vi "Magnetic_Scale_Writing.vi"() -> ()   [LabVIEW 2013]
uses:
  <vilib>/event_ctls.llb/eventvkey.ctl
  Global_Not-Aus.vi
  Global_Start_Stop_Einzelschritt.vi
  <vilib>/Utility/file.llb/Write To Spreadsheet File (DBL).vi
  <vilib>/Instr/_visa.llb/VISA Configure Serial Port (Instr).vi
  <vilib>/Utility/file.llb/Read From Spreadsheet File (string).vi
panel:
  in  "RON settings":T1={"RON Affected axes"=[], "Reference mode"=[], "Check FRF?"=TRUE}
  out "error out 8":errorcluster
  out "error out 4":errorcluster
  out "read buffer":string
  out "error out 7":errorcluster
  out "error out 6":errorcluster
  out "error out 5":errorcluster
  in  "error in 4":errorcluster
  in  "write buffer":string="raw_alls"
  in  "Schritte oder mm (mm)":u16(ring) items=["Schritte", "mm"]
  in  "write ED33 2":string="z\\r"
  in  "write ED33":string="Z\\r"
  out "Diff":i64
  out "Ref_Steps":i64
  out "ED33_pos":i64
  out "ED33_array":string[](array[string])
  out "error out 3":errorcluster
  out "error out 2":errorcluster
  out "error out":errorcluster
  in  "error in":errorcluster
  in  "Tab Control":enum32{"Page 2"}(tab)
  in  "Main Tab":enum32{"Page 1", "Page 2"}(tab)
  out "SensorStage - Zaxis":dbl[](array[numeric]) format="%.6f"
  out "Steps":dbl
  out "Current Sequence":string[](array[string])
  in  "Clear Sequence":bool
  in  "Load Sequence":bool
  out "Sequence":string[][](array[string])
  in  "File  Select":path
  in  "Activate Sequence?":bool
  in  "Multiple Control":T2(tab)
  out "P6":dbl[](array[numeric])
  out "P5":dbl[](array[numeric])
  out "P4":dbl[](array[numeric])
  out "P3":dbl[](array[numeric])
  out "P7":dbl[](array[numeric])
  out "P2":dbl[](array[numeric])
  out "P1":dbl[](array[numeric])
  out "P8":dbl[](array[numeric])
  out "P9":dbl[](array[numeric])
  out "P10":dbl[](array[numeric])
  in  "Z axis":enum16{"Up", "Down"}(ring)
  in  "Y axis":enum16{"Forward", "Backward"}(ring)
  in  "X axis":enum16{"Left", "Right"}(ring)
  in  "Move Steps":bool
  in  "Steps(mm)":dbl[](array[numeric]) min=0.0
  in  "Go To":bool
  in  "Position":T3(ring)
  in  "Save":bool
  in  "Reset All":bool
  in  "Reset":bool
  in  "Import":bool
  in  "Export":bool
  in  "File Path":path=path "Y:/01_Projekte/EPN93031_Schreibplatz/8_Konstruktionsunterlagen/8.5_Software/COPY_KOSY Steuerung LabVIEW/1.New_Code_2014_2015/New_Scripts/1Poletab_position_Ghead.txt"
  out "Speed":dbl(knob) scale=0.0..10.0
  in  "Port for KOSY3":refnum<visa-resource-name>="COM2"
  in  "Port for Powersupply":refnum<visa-resource-name>="COM3"
  in  "Port for Write Head":refnum<visa-resource-name>="COM4"
  in  "Port for ED33":refnum<visa-resource-name>="COM7"
  in  "Port for Sensors":refnum<visa-resource-name>="COM6"
  in  "X,Y,Z Value Limits":T4={"mm Xmin "=0.0, "mm Xmax "=100.0, " mm Ymin "=0.0, "mm Ymax "=267.9, " mm Zmin"=0.0, "mm Zmax "=108.0, "Schritte oder mm Umin (0)"=0.0, "Schritte oder mm Umax (0)"=0.0, "Schritte oder mm Cmin (0)"=0.0, "Schritte oder mm Cmax (0)"=0.0, "Schritte oder mm Amin (0)"=0.0, "Schritte oder mm Amax (0)"=0.0, "Schritte oder mm Bmin (0)"=0.0, "Schritte oder mm Bmax (0)"=0.0}
  out "Error Out":errorcluster caption="error out"
  in  "Error In":errorcluster caption="error in"
  out "Movement":T5={"Axis"=36, "Direction(To/From)"=0, "Speed in mm/s\n (5)[0,025-20]"=5.0, "IV6"=FALSE} {"Direction(To/From)" items=["vom Endschalter weg", "zum Endschalter hin"]; "Speed in mm/s\n (5)[0,025-20]" min=0.025 max=20; "Axis" items=["X-Achse"=36, "Y-Achse"=37, "Z-Achse"=38, "U-Achse"=63]}
  out "Keyboard Press Display":cluster{"Speed(+/-)":i16, "Movement":T6}
  in  "Y_Axis_Select":string(combo)="PI"
  in  "Read Sensor":bool
  in  "Pole Pitch":string(combo)
  in  "Move WithRef":bool
  in  "Sensor Box":string(combo)="MLS5000"
  in  "Sensors Active?":bool
  in  "ED33 Active?":bool
  out "Sensor":cluster{i32, i32}(graph)
  in  "Count":dbl
  in  "Move & Measure":bool
  in  "Clear Sensor Readings":bool
  out "ED33_output":string[][](array[string])
  out "Sensor_output":string[][](array[string])
  out "ED33":i32[](graph)
  out "Sensor Output":string[](array[string])
  out "current time":timestamp
  in  "Move Rel Y":bool
  in  "Stop YaxisStage":bool caption="Stop Yaxis Stage"
  in  "Position to move-Y":dbl[](array[numeric]) format="%.6f"
  in  "Move Abs Y":bool
  in  "Steps to move-Y":dbl[](array[numeric]) format="%.6f"
  in  "System no.Y":i32=2 min=1 step=1
  in  "Axes to move Y":string[](array[string])=["1"]
  out "Ref. Position Y":dbl[](array[numeric]) format="%.6f"
  out "Serial Number Y":string="0145500519"
  in  "Interface Y":u16(ring)=2 items=["RS232", "RS232 DaisyChain", "USB", "USB_DaisyChain"]
  in  "Stop Sensor Stage":bool
  in  "Move Rel S":bool
  in  "Move Abs S":bool
  in  "System no. S":i32=1 min=1 step=1
  in  "Interface S":u16(ring)=2 items=["RS232", "RS232 DaisyChain", "USB", "USB_DaisyChain"]
  in  "Axes to move S":string[](array[string])=["1"]
  out "Serial Number S":string="0135500035"
  out "Ref. Position S":dbl[](array[numeric]) format="%.6f"
  in  "Position to move-S":dbl[](array[numeric]) format="%.6f"
  in  "Steps to move-S":dbl[](array[numeric]) format="%.6f"
  out "Operation Done":string="Initialise"
  out "Current Status":string="Initialise"
  out "Moving":bool
  out "Stopped":bool
  in  "Stop Program":bool
  in  "Home Position":bool
  out "Current Cordinates":T7 {"Schritte B" format="%#.4g"; "Schritte A" format="%#.4g"; "Schritte C" format="%#.4g"; "Schritte U" format="%#.4g"; "Z axis" format="%#.4g"; "Y axis" format="%#.4g"; "X axis" format="%#.4g"}
  out "Yaxis Stage":dbl[](array[numeric]) format="%.6f"
  # "Instructions\n                                              Manual Control\n1. First run PIMikroMove to reference C-863 motor. \n2. Run the program.\n3. Select 'Initialise' to start the program from first \n     or 'Continue' to continue the ongoing process.\n4. Select 'Normal Operation'.\n\nPolestrip Positions\n1. If positions are already saved, select the corresponding \n    file in 'File Path' and then click 'Import' to get the corresponding\n    positions displayed on the front panel. \n2. Set the 'Speed' using (+/-) for the movement.\n3. Select a position from the dropdown 'Position'and click 'Go To'.\n    Else, \n1. Set the 'Speed' using (+/-) for the movement.\n2. Set the length for movement in 'Steps(mm)'  in corresponding \n    axis and also the direction of travel in the selected axis. \n    Then press 'Move'.\n3. Once desired position is reached, select a position from the \n    dropdown 'Position' and click 'Save'.\n4. Once all positions are saved in front panel, select the file  to be \n     saved in 'File Path' and click 'Export' to save positions to a text file.\n5. Select a position from the dropdown 'Position' and \n    Click 'Reset' to clear individual position.\n6. Click 'Reset All' to clear all positions.\n \nSensor Readings\nContinuous measurement\n1.Activate the sensor to be read from 'Read Sensors' tab.\n2.Set the length for movement in 'Steps(mm)' in corresponding \n    axis and also the direction of travel in the selected axis. \n    Then press 'Move'.\nMove and Measure\n1. Activate the sensor to be read from 'Read Sensors' tab.\n2.Set 'Count' to the number of times to measure.\n2.Set the length for movement in 'Steps(mm)' in corresponding \n    axis and also the direction of travel in the selected axis. \n    Then press 'Move Measure'.\n\n1. Click 'Clear' in 'Read Sensors' tab to clear the sensor readings.\n\n                                          Automatic Execution\n1. First run PIMikroMove to reference C-863 motor. \n2. Run the program.\n3. Select 'Initialise' to start the program from first \n     or 'Continue' to continue the ongoing process.\n4. Select 'Normal Operation'.\n5. Select the corresponding file in 'File Select' and then click 'Load' \n    to get the corresponding codes in 'Sequence' .\n6. Click 'Clear' to clear sequence.\n7. Click 'Activate Sequence?' to run the automatic execution. \n\n                                                       General\n1. Click 'Stop Program' to stop the running program.\n2. Click 'Home Position' to take the write head to (0,0,0)."
  # "Write & Read Apparatus ( Control Panel )"
  # "Polestrip Positions"
  # "Com port info"
  # "Waveform Dispaly"
  # "Stage Move - Abs"
  # "Stage Move - Rel"
  # "Stage Move - Abs"
  # "Stage Move - Rel"
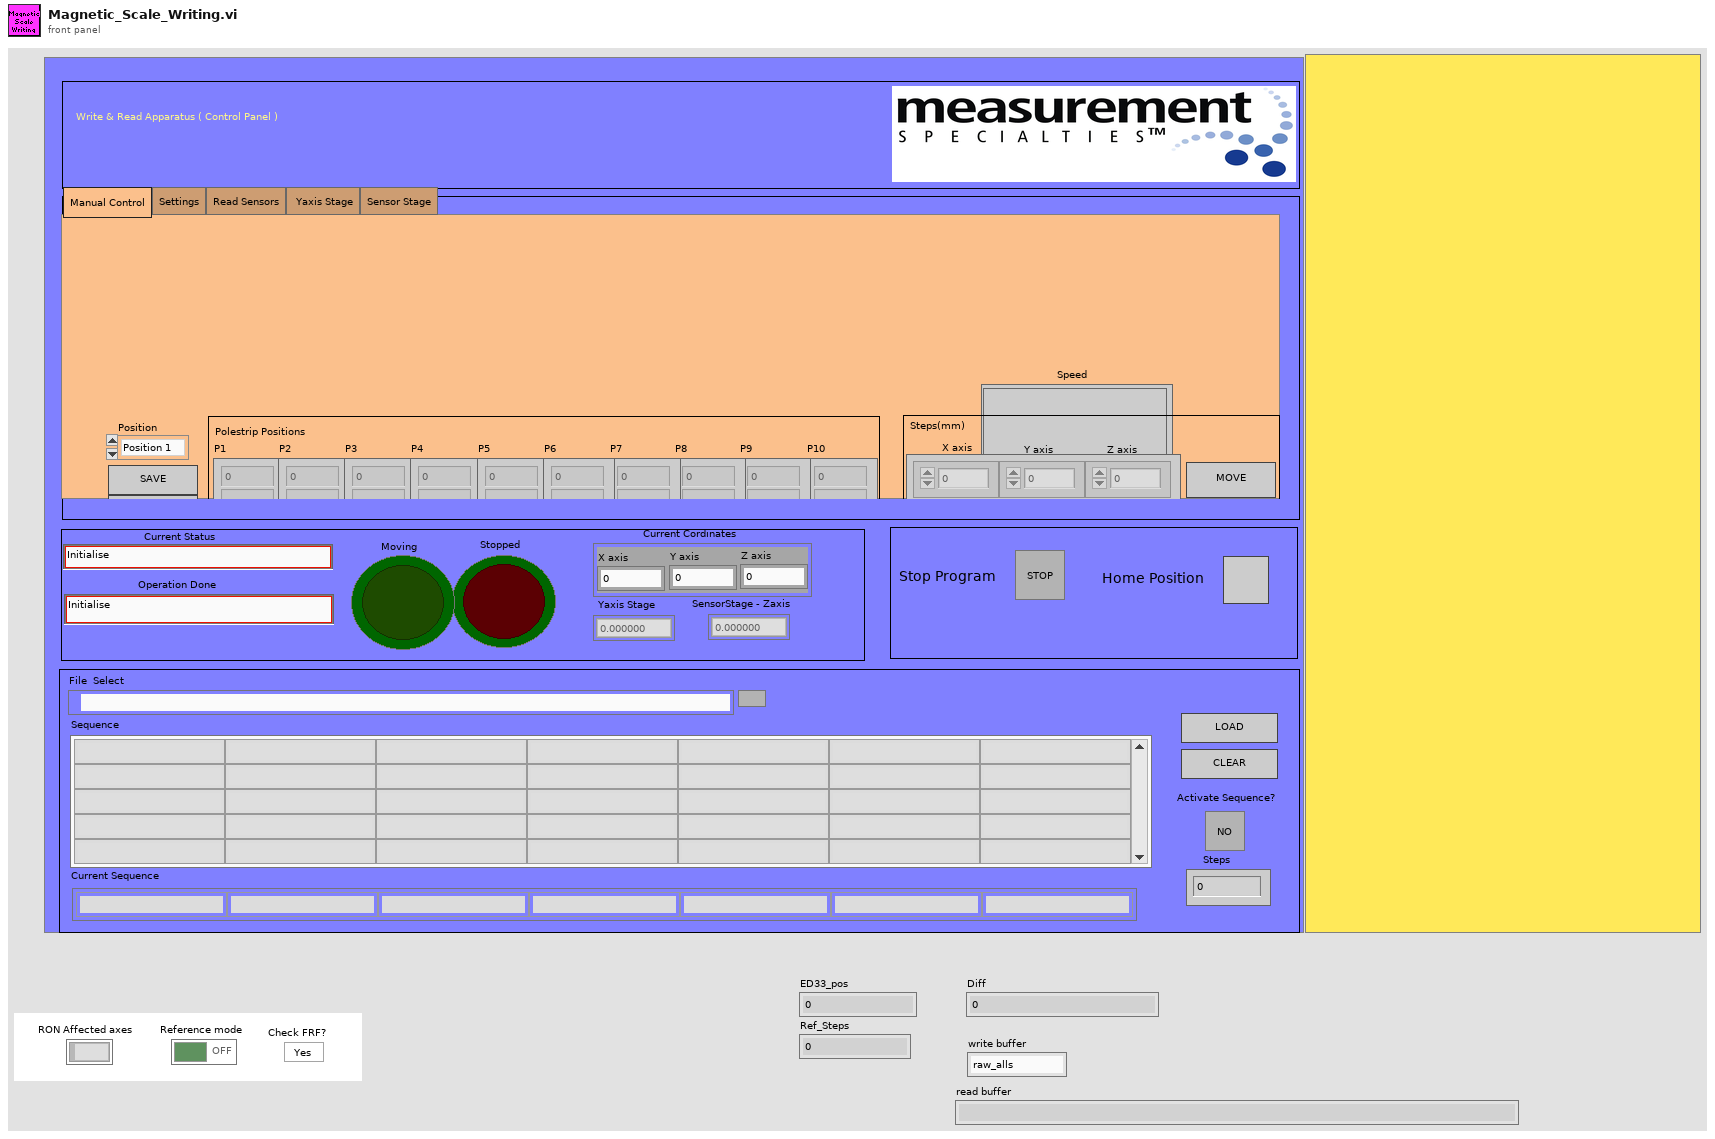
[diagram p1: front panel]
types:
  T1 = cluster{"RON Affected axes":string[], "Reference mode":bool[], "Check FRF?":bool}
  T2 = enum32{"Manual Control", "Settings", "Read Sensors", " Yaxis Stage", "Sensor Stage"}
  T3 = enum16{"Position 1", "Position 2", "Position 3", "Position 4", "Position 5", "Position 6", "Position 7", "Position 8", "Position 9", "Position 10"}
  T4 = cluster{"mm Xmin ":sgl, "mm Xmax ":sgl, " mm Ymin ":sgl, "mm Ymax ":sgl, " mm Zmin":sgl, "mm Zmax ":sgl, "Schritte oder mm Umin (0)":sgl, "Schritte oder mm Umax (0)":sgl, "Schritte oder mm Cmin (0)":sgl, "Schritte oder mm Cmax (0)":sgl, "Schritte oder mm Amin (0)":sgl, "Schritte oder mm Amax (0)":sgl, "Schritte oder mm Bmin (0)":sgl, "Schritte oder mm Bmax (0)":sgl}
  T5 = cluster{"Axis":u8, "Direction(To/From)":u8, "Speed in mm/s\n (5)[0,025-20]":sgl, "IV6":bool}
  T6 = typedef "eventvkey.ctl" = enum16{"ASCII", "Enter", "Return", "Shift", "Ctrl", "Alt", "Cmd", "Opt", "Caps", "NumLock", "Clear", "Break", "Up", "Down", "Left", "Right", "Insert", "Delete", "Home", "End", "PageUp", "PageDown", "Escape", "Help", "Pause", "ScrollLock", "F1", "F2", "F3", "F4", "F5", "F6", "F7", "F8", "F9", "F10", "F11", "F12", "F13", "F14", "F15", "F16", "F17", "F18", "F19", "F20", "F21", "F22", "F23", "F24", "Play", "VolumeUp", "VolumeDown", "Mute", "Two Byte Char"}
  T7 = cluster{"X axis":sgl, "Y axis":sgl, "Z axis":sgl, "Schritte U":sgl, "Schritte C":sgl, "Schritte A":sgl, "Schritte B":sgl}
  T8 = cluster{"Geschwindigkeit X in mm/s\n(5) [0,025-15]":sgl, "Geschwindigkeit Y in mm/s\n(5) [0,025-15]":sgl, "Geschwindigkeit Z in mm/s\n(5) [0,025-15]":sgl, "GeschwindigkeitU in mm/s\n(5) [0,025-15]":sgl}
  T9 = cluster{"Schritte X":sgl, "Schritte Y":sgl, "Schritte Z":sgl, "Schritte U":sgl, "Schritte C":sgl, "Schritte A":sgl, "Schritte B":sgl}
  T10 = cluster{"[0]":dbl, "[1]":dbl, "[2]":dbl, "[3]":dbl, "[4]":dbl, "[5]":dbl, "[6]":dbl, "[7]":dbl, "[8]":dbl}
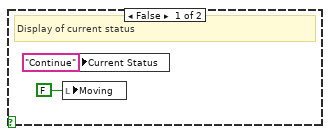
[diagram p5: hidden frame]
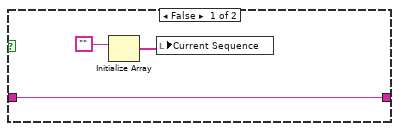
[diagram p6: hidden frame]
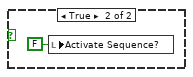
[diagram p7: hidden frame]
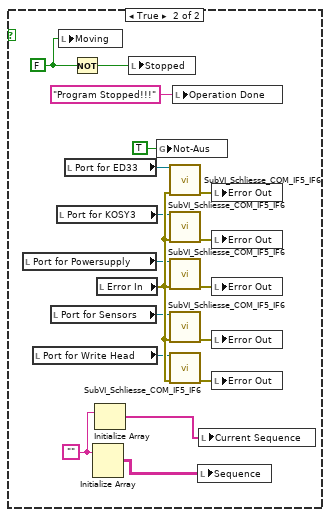
[diagram p8: hidden frame]
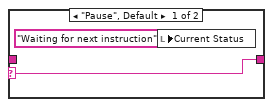
[diagram p9: hidden frame]
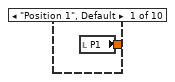
[diagram p11: hidden frame]
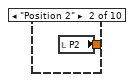
[diagram p12: hidden frame]
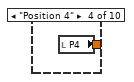
[diagram p13: hidden frame]
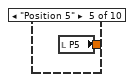
[diagram p14: hidden frame]
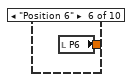
[diagram p15: hidden frame]
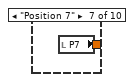
[diagram p16: hidden frame]
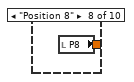
[diagram p17: hidden frame]
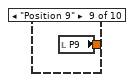
[diagram p18: hidden frame]
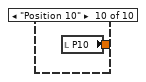
[diagram p19: hidden frame]
diagram:
  n1 = stacked-sequence {
    tunnel: [_ w29] -> w1
    frame #0 {
      w6 = i64 0 ("ED33_pos")
      w8 = 0.0 ("Speed")
      w4 = "" ("element")
      w9 = dbl[] [0.0, 0.0, 0.0] ("P1")
      w2 = FALSE ("Moving")
      # "Start Options - The program starts in this window with an initilialisation. It sets the current status, set all the corresponding booleans to 'False' and the passes on the flow to the next window for further initialisation of the KOSY3 platform and other processes."
      n2 = local read "Error In"() -> (w15:errorcluster)
      n3 = call "Start"("error in (no error)"=w15) -> ("Initialise"=w13:bool, "error out"=w14:errorcluster)  [unwired: 17 in]
      n4 = local write "Error Out"(w14) -> ()
      n5 = case shown="True" w13 {
        frame False {
        }
        frame True {
          n6 = local read "Port for KOSY3"() -> (w18:refnum<visa-resource-name>)
          n7 = local read "Error In"() -> (w17:errorcluster)
          n8 = call "SubVI_Schliesse_COM_IF5_IF6.vi"("VISA resource name in"=w18, "error in"=w17) -> ("error out"=w16:errorcluster)  [unwired: 13 in]
          n9 = local write "Error Out"(w16) -> ()
        }
      }
      n10 = case shown="True" w13 {
        frame False {
          # "Display of current status"
          n11 = local write "Moving"(FALSE ("Stopped")) -> ()
          n12 = local write "Current Status"("Continue") -> ()
        }
        frame True {
          w26 = FALSE ("Stopped")
          # "Display of current status"
          n13 = local write "Current Status"("Initialise") -> ()
          n14 = local write "Stopped"(w26) -> ()
          n15 = Not(x=w26) -> (.not. x?=w27:bool)
          n16 = local write "Moving"(w27) -> ()
        }
      }
      n17 = case shown="True" w13 {
        frame False {
        }
        frame True {
          w22 = u16 0 items=["vom Endschalter weg", "zum Endschalter hin"]
          w23 = u16 36 items=["x-axis"=36, "y-axis"=37, "z-axis"=38]
          # "Initialy setting the boolean in the cluster to False"
          n18 = Bundle(w23, w22, 0.0, FALSE) -> (w19:cluster{u16, u16, dbl, bool})  [unwired: 1 in]
          n19 = local write "Movement"(w19) -> ()
        }
      }
      n20 = local write "Steps(mm)"(w9) -> ()
      n21 = local write "Save"(w2) -> ()
      n22 = local write "Reset"(w2) -> ()
      n23 = local write "Go To"(w2) -> ()
      n24 = local write "Export"(w2) -> ()
      n25 = local write "Move Abs S"(w2) -> ()
      n26 = local write "Move Rel S"(w2) -> ()
      n27 = local write "Stop YaxisStage"(w2) -> ()
      n28 = local write "Move Abs Y"(w2) -> ()
      n29 = local write "Move Rel Y"(w2) -> ()
      n30 = global write "Global_Not-Aus.vi" "Not-Aus"(w2) -> ()
      n31 = local write "Stop Program"(w2) -> ()
      n32 = local write "Stopped"(w2) -> ()
      n33 = local write "Moving"(w2) -> ()
      n34 = local write "Load Sequence"(w2) -> ()
      n35 = local write "Clear Sequence"(w2) -> ()
      n36 = local write "Activate Sequence?"(w2) -> ()
      n37 = local write "Reset All"(w2) -> ()
      n38 = local write "Move WithRef"(w2) -> ()
      n39 = local write "Import"(w2) -> ()
      n40 = local write "Move Steps"(w2) -> ()
      n41 = local write "Sensors Active?"(w2) -> ()
      n42 = local write "ED33 Active?"(w2) -> ()
      n43 = local write "Clear Sensor Readings"(w2) -> ()
      n44 = local write "Move & Measure"(w2) -> ()
      n45 = local write "Stop Sensor Stage"(w2) -> ()
      n46 = local write "Read Sensor"(w2) -> ()
      n47 = Initialize Array(w4) -> (→"Sequence" →"Sensor_output" →"ED33_output":string[][])  [unwired: 2 in]
      n48 = Initialize Array(w4) -> (w3:string[])  [unwired: 1 in]
      n49 = local write "Sensor Output"(w3) -> ()
      n50 = local write "Count"(w8) -> ()
      n51 = property on="ED33" class="WFChart (strict)"("History Data"=i32[] []) -> ()  [unwired: 2 in, 2 out]
      n52 = property on="Sensor" class="WFChart (strict)"("History Data"=cluster{i32, i32}[] []) -> ()  [unwired: 2 in, 2 out]
      "Speed" <- w8
      "P1" <- w9
      "P2" <- w9
      "P3" <- w9
      "P7" <- w9
      "P4" <- w9
      "P5" <- w9
      "P6" <- w9
      "P8" <- w9
      "P9" <- w9
      "P10" <- w9
      "Current Sequence" <- string[] [] ("Current Sequence")
      "Operation Done" <- "Waiting for next instruction" ("Operation Done")
      "Steps" <- w8
      "Diff" <- w6
      "Ref_Steps" <- w6
      "ED33_pos" <- w6
    }
    frame #1 {
      n53 = while {
        stop <- w1640 stop-if-true
        n54 = event shown="[14] \"Stop YaxisStage\": Value Change" {
          selector: _ -> [_ _ _ _ _ _ _ _ _ _ _ _ _ _ _ _ _ _ _ _ _]
          dyn-events: _ -> [_ _ _ _ _ _ _ _ _ _ _ _ _ _ _ _ _ _ _ _ _]
          timeout: 50 -> [_ _ _ _ _ _ _ _ _ _ _ _ _ _ _ _ _ _ _ _ _]
          event Timeout {
            n55 = event-data() -> ()  [unwired: 1 in, 2 out]
            n56 = global write "Global_Start_Stop_Einzelschritt.vi" "Boolesch"(FALSE ("Boolesch")) -> ()
          }
          event Key Down? {
            # "This window checks for the key press in key board. Upon detection, it would set speed and (or) movement cluster and also updates the status."
            n57 = event-data() -> ("Char"=w1643:i16, "VKey"=w1645:T6)  [unwired: 1 in, 8 out]
            n58 = Wait (ms)(milliseconds to wait=u32 200) -> ()  [unwired: 1 out]
            n59 = Bundle("Char"=w1643, "VKey"=w1645) -> (→"Keyboard Press Display":cluster{"Char":i16, "VKey":T6})  [unwired: 1 in]
            n60 = local read "Moving"() -> (w1647:bool)
            n61 = case shown="False" w1647 {
              tunnel: w1645 -> [w1653 _]
              tunnel: w1643 -> [w1655 _]
              frame False {
                n62 = case shown="\"Return\", Default" w1653 {
                  tunnel: [w1656 w1659 w1662 w1665 w1668 w1671 FALSE] -> w1652
                  tunnel: [w1658 w1661 w1664 w1667 w1670 w1673 _] -> w1650
                  tunnel: [w1657 w1660 w1663 w1666 w1669 w1672 _] -> w1649
                  tunnel: TRUE -> [w1656 w1659 w1662 w1665 w1668 w1671 _]
                  frame "Left" {
                    w1657 = u16 1 items=["vom Endschalter weg", "zum Endschalter hin"]
                    w1658 = u16 36 items=["x-axis"=36, "y-axis"=37, "z-axis"=38]
                    # "Direction control(VKey identifies the directional keys)"
                  }
                  frame "Right" {
                    w1660 = u16 0 items=["vom Endschalter weg", "zum Endschalter hin"]
                    w1661 = u16 36 items=["x-axis"=36, "y-axis"=37, "z-axis"=38]
                    # "Direction control"
                  }
                  frame "Up" {
                    w1663 = u16 1 items=["vom Endschalter weg", "zum Endschalter hin"]
                    w1664 = u16 37 items=["x-axis"=36, "y-axis"=37, "z-axis"=38]
                    # "Direction control"
                  }
                  frame "Down" {
                    w1666 = u16 0 items=["vom Endschalter weg", "zum Endschalter hin"]
                    w1667 = u16 37 items=["x-axis"=36, "y-axis"=37, "z-axis"=38]
                  }
                  frame "PageUp" {
                    w1669 = u16 1 items=["vom Endschalter weg", "zum Endschalter hin"]
                    w1670 = u16 38 items=["x-axis"=36, "y-axis"=37, "z-axis"=38]
                  }
                  frame "PageDown" {
                    w1672 = u16 0 items=["vom Endschalter weg", "zum Endschalter hin"]
                    w1673 = u16 38 items=["x-axis"=36, "y-axis"=37, "z-axis"=38]
                  }
                  frame "Return", Default {
                  }
                }
                n63 = local read "Speed"() -> (w1648:dbl)
                n64 = call "Speed_set.vi"("Speed"=w1648, "Char"=w1655) -> ("Speed"=w1654:dbl)
                n65 = local write "Speed"(w1654) -> ()
                n66 = case shown="True" w1652 {
                  tunnel: w1654 -> [_ w1678]
                  tunnel: w1650 -> [_ w1677]
                  tunnel: w1649 -> [_ w1676]
                  frame False {
                  }
                  frame True {
                    n67 = Bundle(w1677, w1676, "Speed"=w1678, TRUE) -> (w1675:cluster{u16, u16, "Speed":dbl, bool})  [unwired: 1 in]
                    n68 = local write "Movement"(w1675) -> ()
                    n69 = local write "Current Status"("Manual Control" ("Status")) -> ()
                  }
                }
              }
              frame True {
                n70 = global write "Global_Start_Stop_Einzelschritt.vi" "Boolesch"(TRUE) -> ()
                n71 = local write "Moving"(FALSE) -> ()
              }
            }
            n72 = event-data() -> ()  [unwired: 3 in, 1 out]
          }
          event "Home Position": Value Change {
            # "This window corresponds to the 'Home position' button on the Front Panel. Pressing the button will take KOSY3 paltform to the home position (0,0,0)"
            n73 = event-data() -> ()  [unwired: 1 in, 6 out]
            n74 = local write "Current Status"("Home Position" ("Status")) -> ()
          }
          event "Save": Value Change {
            # "When the 'SAVE' button in the Front Panel is pressed, it would save the current cordinates of the KOSY3 platform to the selected position."
            n75 = event-data() -> ()  [unwired: 1 in, 6 out]
            n76 = local write "Current Status"("Save Positions" ("Status")) -> ()
          }
          event "Reset": Value Change {
            # "When 'RESET' in the Front Panel is pressed, it resets the cordinates in the selected position to (0,0,0)"
            n77 = event-data() -> ()  [unwired: 1 in, 6 out]
            n78 = local write "Current Status"("Reset Position" ("Status")) -> ()
          }
          event "Reset All": Value Change {
            # "When 'RESET ALL' in the Front Panel is pressed, it resets the cordinates in all positions to (0,0,0)"
            n79 = event-data() -> ()  [unwired: 1 in, 6 out]
            n80 = local write "Current Status"("Reset All" ("Status")) -> ()
          }
          event "Go To": Value Change {
            n81 = event-data() -> ()  [unwired: 1 in, 6 out]
            n82 = local write "Current Status"("Go Position" ("Status")) -> ()
          }
          event "Move Steps": Value Change {
            n83 = event-data() -> ()  [unwired: 1 in, 6 out]
            n84 = local write "Current Status"("Go Straight" ("Status")) -> ()
          }
          event "Move & Measure": Value Change {
            n85 = event-data() -> ()  [unwired: 1 in, 6 out]
            n86 = local write "Current Status"("Move & Measure" ("Status")) -> ()
          }
          event "Move Abs Y": Value Change {
            n87 = event-data() -> ()  [unwired: 1 in, 6 out]
            n88 = local write "Current Status"("YaxisStage Move" ("Current Status")) -> ()
          }
          event "Move Rel Y": Value Change {
            n89 = event-data() -> ()  [unwired: 1 in, 6 out]
            n90 = local write "Current Status"("YaxisStage Move" ("Current Status")) -> ()
          }
          event "Move Abs S": Value Change {
            n91 = event-data() -> ()  [unwired: 1 in, 6 out]
            n92 = local write "Current Status"("SensStage Move" ("Current Status")) -> ()
          }
          event "Move Rel S": Value Change {
            n93 = event-data() -> ()  [unwired: 1 in, 6 out]
            n94 = local write "Current Status"("SensStage Move" ("Current Status")) -> ()
          }
          event "Stop Sensor Stage": Value Change {
            n95 = event-data() -> ()  [unwired: 1 in, 6 out]
            n96 = flat-sequence {
              frame #0 {
                n97 = call "STP.vi"("System no."=2, "All axes?"=TRUE) -> ()  [unwired: 17 in, 1 out]
              }
              frame #1 {
                n98 = local write "Stop Sensor Stage"(FALSE ("Stop Sensor Stage")) -> ()
              }
            }
          }
          event "Stop YaxisStage": Value Change {
            n99 = event-data() -> ()  [unwired: 1 in, 6 out]
            n100 = flat-sequence {
              frame #0 {
                n101 = call "STP.vi"("System no."=1, "All axes?"=TRUE) -> ()  [unwired: 17 in, 1 out]
              }
              frame #1 {
                n102 = local write "Stop YaxisStage"(FALSE ("Stop")) -> ()
              }
            }
          }
          event "Import": Value Change {
            n103 = event-data() -> ()  [unwired: 1 in, 6 out]
            n104 = local write "Current Status"("Import Cordinates" ("Status")) -> ()
          }
          event "Export": Value Change {
            n105 = event-data() -> ()  [unwired: 1 in, 6 out]
            n106 = local write "Current Status"("Export Cordinates" ("Status")) -> ()
          }
          event "Load Sequence": Value Change {
            n107 = event-data() -> ()  [unwired: 1 in, 6 out]
            n108 = local write "Current Status"("Load Sequence" ("Status")) -> ()
          }
          event "Clear Sequence": Value Change {
            n109 = event-data() -> ()  [unwired: 1 in, 6 out]
            n110 = local write "Current Status"("Clear Sequence" ("Status")) -> ()
          }
          event "Clear Sensor Readings": Value Change {
            n111 = event-data() -> ()  [unwired: 1 in, 6 out]
            n112 = local write "Current Status"("Clear SensorReadings" ("Status")) -> ()
          }
          event "Read Sensor": Value Change {
            n113 = event-data() -> ()  [unwired: 1 in, 6 out]
            n114 = local write "Current Status"("Read Sensors" ("Current Status")) -> ()
          }
        }
        n115 = local read "Stop Program"() -> (w1640:bool)
        n116 = global write "Global_Not-Aus.vi" "Not-Aus"(w1640) -> ()
      }
      n117 = local read "Port for KOSY3"() -> (w30:refnum<visa-resource-name>)
      n118 = local read "Current Status"() -> (w32:string)
      n119 = local read "Error In"() -> (w31:errorcluster)
      n120 = while {
        shift-right: [w37] -> w29
        shift-left: w31 -> [w42]
        shift-right: [w38] -> _
        shift-left: w30 -> [w39]
        shift-right: [w40] -> _
        shift-left: w32 -> [w36]
        stop <- w33 stop-if-true
        n121 = local read "Activate Sequence?"() -> (w34:bool)
        n122 = case shown="True" w34 {
          tunnel: w36 -> [w45 _]
          tunnel: [w45 w50] -> w35
          frame False {
            n123 = Initialize Array("") -> (w43:string[])  [unwired: 1 in]
            n124 = local write "Current Sequence"(w43) -> ()
          }
          frame True {
            n125 = local read "Sequence"() -> (w55:string[][])
            n126 = local read "Steps"() -> (w47:dbl)
            n127 = Delete From Array(array=w55, index (row)=0) -> (deleted portion=w52:string[], array with subset deleted=w53:string[][])  [unwired: 2 in]
            n128 = Increment(x=w47) -> (x+1=w46:dbl)
            n129 = local write "Steps"(w46) -> ()
            n130 = local write "Current Sequence"(w52) -> ()
            n131 = Index Array(array=w52, index=0) -> (element=w50:string)
            n132 = Equal?(x=w50, y="Sequence Stop") -> (x = y?=w48:bool)
            n133 = case shown="False" w48 {
              frame False {
              }
              frame True {
                n134 = local write "Activate Sequence?"(FALSE ("Activate Sequence?")) -> ()
              }
            }
            n135 = local write "Sequence"(w53) -> ()
          }
        }
        n136 = case shown="No Error" w42 {
          selector: w42 -> [w83 w1635]
          tunnel: w35 -> [w86 _]
          tunnel: [w85 "Error" ("String 2")] -> w41
          tunnel: w39 -> [w84 w1636]
          tunnel: [w81 w1636] -> w38
          tunnel: [w82 w1635] -> w37
          frame No Error {
            n137 = case shown="\"Move & Measure\"" w86 {
              selector: w86 -> [_ _ _ _ _ _ _ _ _ w480 _ _ _ _ _ _ _ _ _ _ _ _ _ _ _ _ w1625 _]
              tunnel: ["Wait" ("String 2") "Wait" ("String 2") "Wait" ("String 2") "Wait" ("String 2") "Wait" ("String 2") "Wait" ("String 2") "Wait" ("String 2") "Wait" ("String 2") "Wait" ("String 2") w467 "Wait" ("String 2") "Wait" ("String 2") "Wait" "Wait" ("String 2") "Wait" ("String 2") "Wait" ("String 2") "Wait" ("String 2") "Wait" ("String 2") "Wait" ("String 2") "Wait" ("String 2") "Wait" ("String 2") "Wait" ("String 2") "Wait" ("String 2") "Wait" ("String 2") "Wait" ("String 2") "wait" ("String 2") w1625 "Wait" ("String 2")] -> w85
              tunnel: w84 -> [w93 w133 w141 w150 w156 w157 w199 w245 w414 w476 w599 w615 w633 w677 w962 w1127 w1144 w1152 w1179 w1200 w1209 w1225 w1232 w1261 w1269 w1446 w1622 w1627]
              tunnel: w83 -> [w94 w132 w142 w149 w155 w158 w198 w246 w416 w477 w600 w616 w630 w681 w959 w1126 w1143 w1151 w1178 w1201 w1208 w1224 w1230 w1260 w1268 w1442 w1623 w1629]
              tunnel: [w90 w132 w142 w149 w155 w158 w196 w244 w412 w463 w600 w616 w622 w681 w957 w1126 w1143 w1151 w1178 w1201 w1208 w1224 w1230 w1260 w1268 w1442 w1623 w1628] -> w82
              tunnel: [w91 w133 w141 w150 w156 w157 w197 w243 w413 w466 w599 w615 w623 w676 w960 w1127 w1144 w1152 w1179 w1200 w1209 w1225 w1232 w1261 w1269 w1446 w1622 w1627] -> w81
              frame "Batch Position" {
                n138 = flat-sequence {
                  tunnel: w94 -> [w99]
                  tunnel: w93 -> [w98]
                  tunnel: [w97] -> w92
                  tunnel: [w96] -> w89
                  tunnel: w92 -> [w127]
                  tunnel: w89 -> [w126]
                  tunnel: [w127] -> w88
                  tunnel: [w126] -> w87
                  tunnel: [w129] -> w90
                  tunnel: [w130] -> w91
                  tunnel: w88 -> [w130]
                  tunnel: w87 -> [w129]
                  frame #0 {
                    n139 = local read "Current Sequence"() -> (w100:string[])
                    n140 = Index Array(array=w100, index=1) -> (element=w102:string)
                    n141 = case shown="\"Position 3\"" w102 {
                      tunnel: [w110 w111 w112 w113 w114 w115 w116 w117 w118 w119] -> w103
                      frame "Position 1", Default {
                        n142 = local read "P1"() -> (w110:dbl[])
                      }
                      frame "Position 2" {
                        n143 = local read "P2"() -> (w111:dbl[])
                      }
                      frame "Position 3" {
                        n144 = local read "P3"() -> (w112:dbl[])
                      }
                      frame "Position 4" {
                        n145 = local read "P4"() -> (w113:dbl[])
                      }
                      frame "Position 5" {
                        n146 = local read "P5"() -> (w114:dbl[])
                      }
                      frame "Position 6" {
                        n147 = local read "P6"() -> (w115:dbl[])
                      }
                      frame "Position 7" {
                        n148 = local read "P7"() -> (w116:dbl[])
                      }
                      frame "Position 8" {
                        n149 = local read "P8"() -> (w117:dbl[])
                      }
                      frame "Position 9" {
                        n150 = local read "P9"() -> (w118:dbl[])
                      }
                      frame "Position 10" {
                        n151 = local read "P10"() -> (w119:dbl[])
                      }
                    }
                    n152 = local read "Current Cordinates"() -> (w104:T7)
                    n153 = local read "Speed"() -> (w108:dbl)
                    n154 = Bundle(1, "Speed"=w108, 1) -> (w109:cluster{i32, "Speed":dbl, i32})  [unwired: 1 in]
                    n155 = call <userlib>:"SubVI_Punkt_anfahren_IF5_IF6.vi"("Angehängtes Array"=w103, "error in"=w99, "Koordinaten in IF6"=w104, "Geschwindigkeiten"=w109, "VISA resource name in"=w98) -> ("error out"=w96:errorcluster, "Koordinaten out IF6"=w105:T9, "VISA resource name in 2"=w97:refnum<visa-resource-name>)  [unwired: 1 in]
                    n156 = local write "Current Cordinates"(w105) -> ()
                  }
                  frame #1 {
                    w124 = FALSE ("Sensors Active?")
                    n157 = local read "Port for ED33"() -> (w122:refnum<visa-resource-name>)
                    n158 = Not(x=w124) -> (.not. x?=w123:bool)
                    n159 = call "Sensor_Read.vi"("Sensors Active?"=w124, "ED33 Active?"=w123, "Port ED33"=w122) -> ("ED33_output"=w121:string[][])  [unwired: 7 in, 1 out]
                    n160 = Index Array(array=w121, index (row)=0 ("disabled index (col)")) -> (element=w125:string[])  [unwired: 1 in]
                    n161 = local write "Sensor Output"(w125) -> ()
                  }
                  frame #2 {
                    n162 = local write "Operation Done"("Position Set") -> ()
                  }
                }
              }
              frame "Clear SensorReadings" {
                n163 = flat-sequence {
                  frame #0 {
                    n164 = property on="ED33" class="WFChart (strict)"("History Data"=i32[] []) -> ()  [unwired: 2 in, 2 out]
                    n165 = property on="Sensor" class="WFChart (strict)"("History Data"=cluster{"Array 4[0]":i32, "Array 4[1]":i32}[] []) -> ()  [unwired: 2 in, 2 out]
                    n166 = Initialize Array("" ("element")) -> (w135:string[][])  [unwired: 2 in]
                    n167 = call "Sensor_Read.vi"("Clear"=TRUE) -> ()  [unwired: 9 in, 2 out]
                    n168 = local write "Sensor_output"(w135) -> ()
                    n169 = local write "ED33_output"(w135) -> ()
                  }
                  frame #1 {
                    n170 = local write "Clear Sensor Readings"(FALSE ("Clear Sensor Readings")) -> ()
                    n171 = local write "Operation Done"("Cleared sensor readings" ("Operation Done")) -> ()
                  }
                }
              }
              frame "Clear Sequence" {
                n172 = flat-sequence {
                  frame #0 {
                    n173 = Initialize Array("" ("element")) -> (w144:string[][])  [unwired: 2 in]
                    n174 = local write "Sequence"(w144) -> ()
                  }
                  frame #1 {
                    n175 = local write "Clear Sequence"(FALSE ("Clear Sequence")) -> ()
                    n176 = local write "Operation Done"("Sequence cleared" ("Status")) -> ()
                  }
                }
              }
              frame "Display" {
                n177 = One Button Dialog(message="change", button name ("OK")="ok") -> ()  [unwired: 1 out]
              }
              frame "Continue" {
                # "Set the minimum and maximum limits\nfor each axes."
                n178 = local write "X,Y,Z Value Limits"(T4 {"mm Xmin "=0.0, "mm Xmax "=250.0, " mm Ymin "=0.0, "mm Ymax "=267.9, " mm Zmin"=0.0, "mm Zmax "=78.5, "Schritte oder mm Umin (0)"=0.0, "Schritte oder mm Umax (0)"=0.0, "Schritte oder mm Cmin (0)"=0.0, "Schritte oder mm Cmax (0)"=0.0, "Schritte oder mm Amin (0)"=0.0, "Schritte oder mm Amax (0)"=0.0, "Schritte oder mm Bmin (0)"=0.0, "Schritte oder mm Bmax (0)"=0.0} ("X,Y,Z Value Limits")) -> ()
              }
              frame "Export Cordinates" {
                n179 = flat-sequence {
                  frame #0 {
                    n180 = Two Button Dialog(message="Copy the values to ? ", 1:"New File" ("F button name (\"Cancel\")"), 2:"Existing File" ("T button name (\"OK\")")) -> (T button?=w160:bool)
                    n181 = case shown="True" w160 {
                      frame False {
                        n182 = local read "P10"() -> (w170:dbl[])
                        n183 = local read "P1"() -> (w176:dbl[])
                        n184 = local read "P2"() -> (w175:dbl[])
                        n185 = local read "P3"() -> (w174:dbl[])
                        n186 = local read "P4"() -> (w173:dbl[])
                        n187 = local read "P5"() -> (w172:dbl[])
                        n188 = local read "P6"() -> (w171:dbl[])
                        n189 = local read "P7"() -> (w167:dbl[])
                        n190 = local read "P8"() -> (w168:dbl[])
                        n191 = local read "P9"() -> (w169:dbl[])
                        n192 = Build Array(w176, w175, w174, w173, w172, w171, w167, w168, w169, w170) -> (w164:dbl[][])
                        n193 = call-poly <vilib>:"Write To Spreadsheet File.vi"("format (%.3f)"="%.6f", "2D data"=w164) -> ("new file path (Not A Path if cancelled)"=w166:path)  [unwired: 6 in]
                        n194 = local write "File Path"(w166) -> ()
                      }
                      frame True {
                        n195 = local read "P10"() -> (w178:dbl[])
                        n196 = local read "P1"() -> (w179:dbl[])
                        n197 = local read "P2"() -> (w180:dbl[])
                        n198 = local read "P3"() -> (w181:dbl[])
                        n199 = local read "P4"() -> (w182:dbl[])
                        n200 = local read "P5"() -> (w183:dbl[])
                        n201 = local read "P6"() -> (w184:dbl[])
                        n202 = local read "P7"() -> (w185:dbl[])
                        n203 = local read "P8"() -> (w186:dbl[])
                        n204 = local read "P8"() -> (w187:dbl[])
                        n205 = Build Array(w179, w180, w181, w182, w183, w184, w185, w186, w187, w178) -> (w188:dbl[][])
                        n206 = local read "File Path"() -> (w177:path)
                        n207 = call-poly <vilib>:"Write To Spreadsheet File.vi"("format (%.3f)"="%.6f", "2D data"=w188, "file path (dialog if empty)"=w177) -> ()  [unwired: 5 in, 1 out]
                      }
                    }
                  }
                  frame #1 {
                    n208 = local write "Export"(FALSE ("Export")) -> ()
                    n209 = local write "Operation Done"("Export the position cordinates" ("Operation Done")) -> ()
                  }
                }
              }
              frame "Go Position" {
                n210 = flat-sequence {
                  tunnel: [w205] -> w195
                  tunnel: [w204] -> w193
                  tunnel: w199 -> [w207]
                  tunnel: w198 -> [w206]
                  tunnel: w195 -> [w233]
                  tunnel: [w233] -> w194
                  tunnel: w193 -> [w232]
                  tunnel: [w232] -> w192
                  tunnel: [w238] -> w196
                  tunnel: [w239] -> w197
                  tunnel: w194 -> [w239]
                  tunnel: w192 -> [w238]
                  frame #0 {
                    w203 = TRUE ("Moving")
                    n211 = local read "Position"() -> (w215:T3)
                    n212 = case shown="\"Position 10\"" w215 {
                      tunnel: [w216 w217 w218 w219 w220 w221 w222 w223 w224 w225] -> w213
                      frame "Position 1", Default {
                        n213 = local read "P1"() -> (w216:dbl[])
                      }
                      frame "Position 2" {
                        n214 = local read "P2"() -> (w217:dbl[])
                      }
                      frame "Position 3" {
                        n215 = local read "P3"() -> (w218:dbl[])
                      }
                      frame "Position 4" {
                        n216 = local read "P4"() -> (w219:dbl[])
                      }
                      frame "Position 5" {
                        n217 = local read "P5"() -> (w220:dbl[])
                      }
                      frame "Position 6" {
                        n218 = local read "P6"() -> (w221:dbl[])
                      }
                      frame "Position 7" {
                        n219 = local read "P7"() -> (w222:dbl[])
                      }
                      frame "Position 8" {
                        n220 = local read "P8"() -> (w223:dbl[])
                      }
                      frame "Position 9" {
                        n221 = local read "P9"() -> (w224:dbl[])
                      }
                      frame "Position 10" {
                        n222 = local read "P10"() -> (w225:dbl[])
                      }
                    }
                    n223 = local write "ED33 Active?"(TRUE ("ED33 Active?")) -> ()
                    n224 = Not(x=w203) -> (.not. x?=w202:bool)
                    n225 = local write "Moving"(w203) -> ()
                    n226 = local write "Stopped"(w202) -> ()
                    n227 = local read "Current Cordinates"() -> (w212:T7)
                    n228 = local read "Speed"() -> (w209:dbl)
                    n229 = Bundle(0, "Speed"=w209, 0) -> (w208:cluster{i32, "Speed":dbl, i32})  [unwired: 1 in]
                    n230 = call <userlib>:"SubVI_Punkt_anfahren_IF5_IF6.vi"("Angehängtes Array"=w213, "error in"=w206, "Koordinaten in IF6"=w212, "Geschwindigkeiten"=w208, "VISA resource name in"=w207) -> ("error out"=w204:errorcluster, "Koordinaten out IF6"=w214:T9, "VISA resource name in 2"=w205:refnum<visa-resource-name>)  [unwired: 1 in]
                    n231 = local write "Current Cordinates"(w214) -> ()
                  }
                  frame #1 {
                    w231 = FALSE ("Sensors Active?")
                    n232 = local read "Port for ED33"() -> (w226:refnum<visa-resource-name>)
                    n233 = Not(x=w231) -> (.not. x?=w230:bool)
                    n234 = call "Sensor_Read.vi"("Sensors Active?"=w231, "ED33 Active?"=w230, "Port ED33"=w226) -> ("ED33_output"=w229:string[][])  [unwired: 7 in, 1 out]
                    n235 = Index Array(array=w229, index (row)=0 ("disabled index (col)")) -> (element=w227:string[])  [unwired: 1 in]
                    n236 = local write "Sensor Output"(w227) -> ()
                  }
                  frame #2 {
                    w234 = TRUE ("Moving")
                    n237 = local write "Go To"(FALSE ("Go To")) -> ()
                    n238 = local write "Stopped"(w234) -> ()
                    n239 = Not(x=w234) -> (.not. x?=w235:bool)
                    n240 = local write "Moving"(w235) -> ()
                    n241 = local write "Operation Done"("Go to the selected position" ("Operation Done")) -> ()
                  }
                }
              }
              frame "Go Straight" {
                n242 = local read "Sensors Active?"() -> (w240:bool)
                n243 = local read "ED33 Active?"() -> (w241:bool)
                n244 = Or(x=w241, y=w240) -> (x .or. y?=w242:bool)
                n245 = case shown="False" w242 {
                  tunnel: w246 -> [w254 w332]
                  tunnel: w245 -> [w253 w335]
                  tunnel: [w252 w337] -> w244
                  tunnel: [w251 w334] -> w243
                  frame False {
                    n246 = local read "Current Sequence"() -> (w250:string[])
                    n247 = Index Array(array=w250, index=1) -> (element=w248:string)
                    n248 = case shown="\"PI\", Default" w248 {
                      tunnel: w254 -> [w256 w300]
                      tunnel: w253 -> [w257 w299]
                      tunnel: [w255 w298] -> w252
                      tunnel: [w257 w297] -> w251
                      frame "PI", Default {
                        n249 = flat-sequence {
                          tunnel: [w271] -> w266
                          tunnel: [w267] -> w265
                          tunnel: [w270] -> w264
                          tunnel: w256 -> [w268]
                          tunnel: w266 -> [w279]
                          tunnel: w265 -> [w278]
                          tunnel: w264 -> [w282]
                          tunnel: [w280] -> w263
                          tunnel: [w278] -> w262
                          tunnel: [w279] -> w261
                          tunnel: w263 -> [w288]
                          tunnel: [w287] -> w260
                          tunnel: w262 -> [w286]
                          tunnel: [w286] -> w259
                          tunnel: w261 -> [w285]
                          tunnel: [w285] -> w258
                          tunnel: [w294] -> w255
                          tunnel: w260 -> [w292]
                          tunnel: w259 -> [w291]
                          tunnel: w258 -> [w290]
                          frame #0 {
                            n250 = local read "System no.Y"() -> (w267:i32)
                            n251 = local read "Axes to move Y"() -> (w271:string[])
                            n252 = call "VEL.vi"("System no."=w267, "Axes to set"=w271, "Velocity values"=dbl[] [1.0], "error in"=w268) -> ("error out"=w270:errorcluster)  [unwired: 14 in, 1 out]
                          }
                          frame #1 {
                            w274 = 0.0 ("element")
                            n253 = local read "Current Sequence"() -> (w276:string[])
                            n254 = local write "Moving"(TRUE ("Moving")) -> ()
                            n255 = Index Array(array=w276, index=2) -> (element=w275:string)
                            n256 = Fract/Exp String To Number(string=w275) -> (number=w273:dbl)  [unwired: 3 in, 1 out]
                            n257 = Build Array(w273, w274, w274, w274) -> (w272:dbl[])
                            n258 = call "MVR.vi"("System no."=w278, "Axes to move"=w279, "Position values"=w272, "No.of digits"=i16 4, "error in"=w282) -> ("error out"=w280:errorcluster)  [unwired: 14 in]
                          }
                          frame #2 {
                            n259 = call "General wait for movement to stop.vi"("System no."=w286, "Axes to wait for"=w285, "Additional wait time, ms"=u32 500, "error in"=w288) -> ("Stopped"=w284:bool, "error out"=w287:errorcluster)  [unwired: 14 in]
                            n260 = local write "Stopped"(w284) -> ()
                          }
                          frame #3 {
                            n261 = call "POS?.vi"("System no."=w291, "Axes to query"=w290, "error in"=w292) -> ("Position"=w296:dbl[], "error out"=w294:errorcluster)  [unwired: 15 in]
                            n262 = local write "Move Rel Y"(FALSE ("Move Rel")) -> ()
                            n263 = local write "Moving"(FALSE ("Moving")) -> ()
                            n264 = local write "Yaxis Stage"(w296) -> ()
                          }
                        }
                      }
                      frame "KOSY" {
                        n265 = flat-sequence {
                          tunnel: w300 -> [w314]
                          tunnel: [w316] -> w302
                          tunnel: [w315] -> w301
                          tunnel: w299 -> [w313]
                          tunnel: w302 -> [w330]
                          tunnel: [w330] -> w297
                          tunnel: [w329] -> w298
                          tunnel: w301 -> [w329]
                          frame #0 {
                            w320 = TRUE ("Moving")
                            n266 = local read "X axis"() -> (w309:enum16{"Left", "Right"})
                            n267 = local read "Y axis"() -> (w308:enum16{"Forward", "Backward"})
                            n268 = local read "Z axis"() -> (w307:enum16{"Up", "Down"})
                            n269 = Not(x=w320) -> (.not. x?=w319:bool)
                            n270 = local write "Moving"(w320) -> ()
                            n271 = case shown="\"Right\"" w309 {
                              tunnel: [1 0] -> w312
                              frame "Left", Default {
                              }
                              frame "Right" {
                              }
                            }
                            n272 = case shown="\"Forward\", Default" w308 {
                              tunnel: [0 1] -> w311
                              frame "Forward", Default {
                              }
                              frame "Backward" {
                              }
                            }
                            n273 = case shown="\"Down\"" w307 {
                              tunnel: [1 0] -> w310
                              frame "Up", Default {
                              }
                              frame "Down" {
                              }
                            }
                            n274 = local write "Stopped"(w319) -> ()
                            n275 = local read "Steps(mm)"() -> (w306:dbl[])
                            n276 = local read "Activate Sequence?"() -> (w318:bool)
                            n277 = local read "Current Sequence"() -> (w304:string[])
                            n278 = Build Array (concatenate)(w306, w312, w311, w310) -> (w305:dbl[])
                            n279 = local read "Speed"() -> (w303:dbl)
                            n280 = call "Go Straight.vi"("VISA resource name in"=w313, "Sequence Active"=w318, "Current sequence"=w304, "Speed"=w303, "Steps(mm)"=w305, "error in"=w314) -> ("VISA resource name out"=w316:refnum<visa-resource-name>, "Koordinaten IF6"=w317:T9, "error out"=w315:errorcluster)
                            n281 = local write "Current Cordinates"(w317) -> ()
                          }
                          frame #1 {
                            w331 = TRUE ("Stopped")
                            n282 = Not(x=w331) -> (.not. x?=w328:bool)
                            n283 = local write "Stopped"(w331) -> ()
                            n284 = local write "Move Steps"(w328) -> ()
                            n285 = local write "Moving"(w328) -> ()
                            n286 = local write "Operation Done"("Moved to corresponding position" ("Operation Done")) -> ()
                          }
                        }
                      }
                    }
                  }
                  frame True {
                    n287 = flat-sequence {
                      tunnel: w332 -> [w338]
                      frame #0 {
                        n288 = local read "Sensors Active?"() -> (w340:bool)
                        n289 = local read "ED33 Active?"() -> (w339:bool)
                        n290 = case shown="True" w339 {
                          selector: w339 -> [_ w360]
                          tunnel: w338 -> [_ w359]
                          frame False {
                          }
                          frame True {
                            n291 = while {
                              tunnel: w360 -> [w362]
                              tunnel: w359 -> [w369]
                              stop <- w368 stop-if-true
                              n292 = local read "Port for ED33"() -> (w363:refnum<visa-resource-name>)
                              n293 = call "Sensor_Read.vi"("error in (no error)"=w369, "Clear"=FALSE ("ED32i Active?"), "ED33 Active?"=w362, "Port ED33"=w363) -> ("ED33_output"=w365:string[][])  [unwired: 6 in, 1 out]
                              n294 = local write "ED33_output"(w365) -> ()
                              n295 = Index Array(array=w365, index (col)=1) -> (element=w367:string[])  [unwired: 1 in]
                              n296 = local read "Stopped"() -> (w368:bool)
                              n297 = Decimal String To Number(string=w367) -> (number=w364:i32[])  [unwired: 2 in, 1 out]
                              n298 = local write "ED33"(w364) -> ()
                            }
                          }
                        }
                        n299 = case shown="True" w340 {
                          selector: w340 -> [_ w342]
                          tunnel: w338 -> [_ w341]
                          frame False {
                          }
                          frame True {
                            n300 = while {
                              tunnel: w342 -> [w357]
                              tunnel: w341 -> [w356]
                              stop <- w355 stop-if-true
                              n301 = local read "Port for Sensors"() -> (w358:refnum<visa-resource-name>)
                              n302 = call "Sensor_Read.vi"("error in (no error)"=w356, "Clear"=FALSE ("ED33 Active?"), "Sensor Box"="Sensor Box", "Port Sensors"=w358, "Sensors Active?"=w357) -> ("Sensors_output"=w345:string[][])  [unwired: 5 in, 1 out]
                              n303 = local write "Sensor_output"(w345) -> ()
                              n304 = Index Array(array=w345, index (col)=0) -> (element=w352:string[])  [unwired: 1 in]
                              n305 = Index Array(array=w345, index (col)=1) -> (element=w350:string[])  [unwired: 1 in]
                              n306 = Index Array(array=w352) -> (element=w351:string)  [unwired: 1 in]
                              n307 = Index Array(array=w350) -> (element=w349:string)  [unwired: 1 in]
                              n308 = Decimal String To Number(string=w351) -> (number=w348:i32)  [unwired: 2 in, 1 out]
                              n309 = Decimal String To Number(string=w349) -> (number=w347:i32)  [unwired: 2 in, 1 out]
                              n310 = Bundle(w348, w347) -> (w346:cluster{i32, i32})  [unwired: 1 in]
                              n311 = local read "Stopped"() -> (w355:bool)
                              n312 = local write "Sensor"(w346) -> ()
                            }
                          }
                        }
                      }
                      frame #1 {
                        n313 = local read "Current Cordinates"() -> (w374:T7)
                        n314 = local read "Sensors Active?"() -> (w376:bool)
                        n315 = local read "Sensor_output"() -> (w372:string[][])
                        n316 = local read "ED33 Active?"() -> (w375:bool)
                        n317 = local read "ED33_output"() -> (w371:string[][])
                        n318 = local read "Sensor Box"() -> (w370:string)
                        n319 = call "Sensor_Save.vi"("ED33_output"=w371, "Sensor_output"=w372, "ED33 Active?"=w375, "Current Cordinates"=w374, "Sensor Box"=w370, "Cont/MM"="Continuous" ("Movement"), "Sensors Active?"=w376) -> ()  [unwired: 1 in]
                        n320 = local write "Operation Done"("Read values from sensors and values saved" ("Operation Done")) -> ()
                      }
                      frame #2 {
                        w378 = FALSE ("ED32i Active?")
                        n321 = local write "Clear Sensor Readings"(TRUE ("Clear Sensor Readings")) -> ()
                        n322 = local write "ED33 Active?"(w378) -> ()
                        n323 = local write "Sensors Active?"(w378) -> ()
                      }
                    }
                    n324 = flat-sequence {
                      tunnel: w332 -> [w395]
                      tunnel: [w391] -> w336
                      tunnel: w335 -> [w390]
                      tunnel: [w389] -> w333
                      tunnel: [w407] -> w337
                      tunnel: w336 -> [w407]
                      tunnel: [w404] -> w334
                      tunnel: w333 -> [w404]
                      frame #0 {
                        w392 = TRUE ("Moving")
                        n325 = local read "X axis"() -> (w388:enum16{"Left", "Right"})
                        n326 = local read "Y axis"() -> (w387:enum16{"Forward", "Backward"})
                        n327 = local read "Z axis"() -> (w386:enum16{"Up", "Down"})
                        n328 = case shown="\"Right\"" w388 {
                          tunnel: [1 0] -> w384
                          frame "Left", Default {
                          }
                          frame "Right" {
                          }
                        }
                        n329 = case shown="\"Backward\"" w387 {
                          tunnel: [0 1] -> w383
                          frame "Forward", Default {
                          }
                          frame "Backward" {
                          }
                        }
                        n330 = case shown="\"Up\", Default" w386 {
                          tunnel: [1 0] -> w382
                          frame "Up", Default {
                          }
                          frame "Down" {
                          }
                        }
                        n331 = Not(x=w392) -> (.not. x?=w393:bool)
                        n332 = local write "Moving"(w392) -> ()
                        n333 = local write "Stopped"(w393) -> ()
                        n334 = local read "Steps(mm)"() -> (w385:dbl[])
                        n335 = local read "Activate Sequence?"() -> (w396:bool)
                        n336 = local read "Current Sequence"() -> (w397:string[])
                        n337 = Build Array (concatenate)(w385, w384, w383, w382) -> (w381:dbl[])
                        n338 = call "Go Straight.vi"("VISA resource name in"=w390, "Sequence Active"=w396, "Current sequence"=w397, "Speed"=0.025, "Steps(mm)"=w381, "error in"=w395) -> ("VISA resource name out"=w389:refnum<visa-resource-name>, "Koordinaten IF6"=w394:T9, "error out"=w391:errorcluster)
                        n339 = local write "Current Cordinates"(w394) -> ()
                      }
                      frame #1 {
                        w406 = TRUE ("Stopped")
                        n340 = Not(x=w406) -> (.not. x?=w405:bool)
                        n341 = local write "Stopped"(w406) -> ()
                        n342 = local write "Moving"(w405) -> ()
                        n343 = local write "Move Steps"(w405) -> ()
                      }
                    }
                  }
                }
              }
              frame "Home Position" {
                n344 = flat-sequence {
                  tunnel: [w419] -> w417
                  tunnel: w416 -> [w419]
                  tunnel: [w420] -> w415
                  tunnel: w414 -> [w420]
                  tunnel: w417 -> [w424]
                  tunnel: w415 -> [w427]
                  tunnel: [w426] -> w411
                  tunnel: [w423] -> w409
                  tunnel: w411 -> [w433]
                  tunnel: [w433] -> w410
                  tunnel: w409 -> [w432]
                  tunnel: [w431] -> w408
                  tunnel: [w458] -> w413
                  tunnel: w410 -> [w458]
                  tunnel: [w457] -> w412
                  tunnel: w408 -> [w457]
                  frame #0 {
                    w421 = TRUE ("Moving")
                    n345 = Not(x=w421) -> (.not. x?=w422:bool)
                    n346 = local write "Moving"(w421) -> ()
                    n347 = local write "Stopped"(w422) -> ()
                  }
                  frame #1 {
                    w429 = u16 6 items=["X-Achse", "Y-Achse", "Z-Achse", "X- und Y-Achse", "X- und Z-Achse", "Y- und Z-Achse", "X, Y und Z-Achse", "U-Achse", "keine Achse"] ("Beteiligte Achsen (X,Y,Z,U)")
                    n348 = call "SubVI_Home_XYZU_IF5_IF6.vi"("VISA resource name in"=w427, "Beteiligte Achsen (X,Y,Z,U)"=w429, "Geschwindigkeiten"=T8 {"Geschwindigkeit X in mm/s\n(5) [0,025-15]"=10.0, "Geschwindigkeit Y in mm/s\n(5) [0,025-15]"=10.0, "Geschwindigkeit Z in mm/s\n(5) [0,025-15]"=10.0, "GeschwindigkeitU in mm/s\n(5) [0,025-15]"=2.0}, "IF5=F/IF6=T\n(IF6=T) in"=TRUE ("IF5=F/IF6=T\n(IF6=T) in"), "error in"=w424) -> ("VISA resource name out"=w426:refnum<visa-resource-name>, "Koordinaten IF6"=w428:T9, "error out"=w423:errorcluster)  [unwired: 3 in, 5 out]
                    n349 = local write "Current Cordinates"(w428) -> ()
                  }
                  frame #2 {
                    n350 = stacked-sequence {
                      tunnel: w432 -> [w440 w447]
                      tunnel: [w434 _] -> w431
                      frame #0 {
                        n351 = local read "Axes to move Y"() -> (w435:string[])
                        n352 = local read "System no.Y"() -> (w436:i32)
                        n353 = call "VEL.vi"("System no."=w436, "Axes to set"=w435, "Velocity values"=dbl[] [5.9], "error in"=w440) -> ("error out"=w439:errorcluster)  [unwired: 14 in, 1 out]
                        n354 = call "MOV.vi"("System no."=w436, "Axes to move"=w435, "Position values"=dbl[] [21.8], "error in"=w439) -> ("error out"=w438:errorcluster)  [unwired: 15 in]
                        n355 = call "General wait for movement to stop.vi"("System no."=w436, "Axes to wait for"=w435, "Additional wait time, ms"=u32 500, "error in"=w438) -> ("error out"=w437:errorcluster)  [unwired: 14 in, 1 out]
                        n356 = call "POS?.vi"("System no."=w436, "Axes to query"=w435, "All axes?"=TRUE, "error in"=w437) -> ("Position"=w442:dbl[], "error out"=w434:errorcluster)  [unwired: 14 in]
                        n357 = local write "Yaxis Stage"(w442) -> ()
                      }
                      frame #1 {
                        n358 = local read "Axes to move S"() -> (w448:string[])
                        n359 = local read "System no. S"() -> (w449:i32)
                        n360 = call "VEL.vi"("System no."=w449, "Axes to set"=w448, "Velocity values"=dbl[] [2.0], "error in"=w447) -> ("error out"=w452:errorcluster)  [unwired: 14 in, 1 out]
                        n361 = call "FRF.vi"("System no."=w449, "Affected axes"=w448, "error in"=w452) -> ("error out"=w451:errorcluster)  [unwired: 16 in]
                        n362 = call "General wait for movement to stop.vi"("System no."=w449, "Axes to wait for"=w448, "Additional wait time, ms"=u32 500, "error in"=w451) -> ("error out"=w450:errorcluster)  [unwired: 14 in, 1 out]
                        n363 = call "POS?.vi"("System no."=w449, "Axes to query"=w448, "All axes?"=TRUE, "error in"=w450) -> ("Position"=w453:dbl[], "error out"=→"error out 4":errorcluster)  [unwired: 14 in]
                        n364 = local write "SensorStage - Zaxis"(w453) -> ()
                      }
                    }
                  }
                  frame #3 {
                    w461 = FALSE ("Moving")
                    n365 = local write "Home Position"(FALSE ("Go To")) -> ()
                    n366 = Not(x=w461) -> (.not. x?=w462:bool)
                    n367 = local write "Moving"(w461) -> ()
                    n368 = local write "Stopped"(w462) -> ()
                    n369 = local write "Operation Done"("The platform is taken to home position (0,0,0)" ("Operation Done")) -> ()
                  }
                }
              }
              frame "Initialise" {
                n370 = flat-sequence {
                  tunnel: w476 -> [w482]
                  tunnel: w477 -> [w483]
                  tunnel: w480 -> [w484]
                  tunnel: [w484] -> w473
                  tunnel: [w483] -> w472
                  tunnel: [w482] -> w471
                  tunnel: [w491] -> w479
                  tunnel: [w490] -> w478
                  tunnel: [w487] -> w475
                  tunnel: [w486] -> w474
                  tunnel: w473 -> [w492]
                  tunnel: w472 -> [w489]
                  tunnel: w471 -> [w488]
                  tunnel: w479 -> [w496]
                  tunnel: w478 -> [w495]
                  tunnel: w475 -> [w494]
                  tunnel: w474 -> [w493]
                  tunnel: [w495] -> w470
                  tunnel: [w494] -> w469
                  tunnel: [w493] -> w468
                  tunnel: w470 -> [w500]
                  tunnel: w469 -> [w499]
                  tunnel: w468 -> [w497]
                  tunnel: [w500] -> w465
                  tunnel: [w499] -> w464
                  tunnel: [w498] -> w463
                  tunnel: [w544] -> w466
                  tunnel: [w545] -> w467
                  tunnel: w465 -> [w545]
                  tunnel: w464 -> [w544]
                  frame #0 {
                    # "Set the minimum and maximum limits\nfor each axes."
                    n371 = local write "X,Y,Z Value Limits"(T4 {"mm Xmin "=0.0, "mm Xmax "=250.0, " mm Ymin "=0.0, "mm Ymax "=267.9, " mm Zmin"=0.0, "mm Zmax "=78.5, "Schritte oder mm Umin (0)"=0.0, "Schritte oder mm Umax (0)"=0.0, "Schritte oder mm Cmin (0)"=0.0, "Schritte oder mm Cmax (0)"=0.0, "Schritte oder mm Amin (0)"=0.0, "Schritte oder mm Amax (0)"=0.0, "Schritte oder mm Bmin (0)"=0.0, "Schritte oder mm Bmax (0)"=0.0} ("X,Y,Z Value Limits")) -> ()
                  }
                  frame #1 {
                    n372 = local read "X,Y,Z Value Limits"() -> (w485:T4)
                    n373 = call "Initialise.vi"("error IO"=w489, "X,Y,Z values"=w485, "String"=w492, "Port for KOSY3"=w488) -> ("Fehler (Ausgang)"=w486:errorcluster, "Cordinates of the  KOSY3 Platform"=w491:T9, "String 2"=w490:string, "VISA-Referenz (Ausgang)"=w487:refnum<visa-resource-name>)
                  }
                  frame #2 {
                    n374 = local write "Current Cordinates"(w496) -> ()
                  }
                  frame #3 {
                    n375 = stacked-sequence {
                      tunnel: w497 -> [w505 w533]
                      tunnel: [w501 _] -> w498
                      frame #0 {
                        n376 = flat-sequence {
                          tunnel: w505 -> [w507]
                          tunnel: [w506] -> w504
                          tunnel: ["System no.Y"] -> w503
                          tunnel: ["Axes to move Y"] -> w502
                          tunnel: w504 -> [w527]
                          tunnel: w503 -> [w514]
                          tunnel: w502 -> [w515]
                          tunnel: [w513] -> w501
                          frame #0 {
                            n377 = call "VEL.vi"("System no."="System no.Y", "Axes to set"="Axes to move Y", "Velocity values"=dbl[] [5.9], "error in"=w507) -> ("error out"=w506:errorcluster)  [unwired: 14 in, 1 out]
                          }
                          frame #1 {
                            w518 = FALSE ("Stopped")
                            n378 = call "Mercury_GCS_Configuration_Setup.vi"("System no."=w514, "Interface"="Interface Y", "Axes to move"=w515, "error in"=w527, "Switch servo on?"=TRUE) -> ("SN out"=→"Serial Number Y":string, "Position"=→"Ref. Position Y":dbl[], "error out"=w517:errorcluster)  [unwired: 8 in, 4 out]
                            n379 = call "MOV.vi"("System no."=w514, "Axes to move"=w515, "Position values"=dbl[] [21.8], "No.of digits"=i16 4, "error in"=w517) -> ("error out"=w516:errorcluster)  [unwired: 14 in]
                            n380 = call "General wait for movement to stop.vi"("System no."=w514, "Axes to wait for"=w515, "Additional wait time, ms"=u32 500, "error in"=w516) -> ("error out"=w520:errorcluster)  [unwired: 14 in, 1 out]
                            n381 = Not(x=w518) -> (.not. x?=w519:bool)
                            n382 = local write "Moving"(w518) -> ()
                            n383 = call "POS?.vi"("System no."=w514, "Axes to query"=w515, "error in"=w520) -> ("Position"=w524:dbl[], "error out"=w513:errorcluster)  [unwired: 15 in]
                            n384 = local write "Stopped"(w519) -> ()
                            n385 = local write "Yaxis Stage"(w524) -> ()
                          }
                        }
                      }
                      frame #1 {
                        n386 = call "Mercury_GCS_Configuration_Setup.vi"("System no."="System no. S", "RON settings"="RON settings", "Interface"="Interface S", "Axes to move"="Axes to move S", "error in"=w533, "Switch servo on?"=TRUE) -> ("SN out"=→"Serial Number S":string, "Position"=→"Ref. Position S":dbl[], "error out"=w538:errorcluster)  [unwired: 7 in, 4 out]
                        n387 = call "General wait for movement to stop.vi"("System no."="System no. S", "Axes to wait for"="Axes to move S", "Additional wait time, ms"=u32 500, "error in"=w538) -> ("Stopped"=w529:bool, "error out"=w534:errorcluster)  [unwired: 14 in]
                        n388 = local write "Stopped"(w529) -> ()
                        n389 = call "POS?.vi"("System no."="System no. S", "Axes to query"="Axes to move S", "error in"=w534) -> ("Position"=→"SensorStage - Zaxis":dbl[], "error out"=→"error out 8":errorcluster)  [unwired: 15 in]
                      }
                    }
                  }
                  frame #4 {
                    n390 = stacked-sequence {
                      frame #0 {
                        n391 = local read "Port for ED33"() -> (w578:refnum<visa-resource-name>)
                        n392 = call-poly "VISA Configure Serial Port"("VISA resource name"=w578) -> ("VISA resource name out"=w567:refnum<visa-resource-name>, "error out"=w568:errorcluster)  [unwired: 8 in, 5 out]
                        n393 = flat-sequence {
                          tunnel: w569 -> [w580]
                          tunnel: [w580] -> w570
                          tunnel: [w579] -> w571
                          tunnel: w572 -> [w579]
                          frame #0 {
                            n394 = Wait (ms)(milliseconds to wait=u32 100) -> ()  [unwired: 1 out]
                          }
                        }
                        n395 = VISA Write(VISA resource name=w567, write buffer="write ED33", error in (no error)=w568) -> (VISA resource name out=w569:refnum<visa-resource-name>, error out=w572:errorcluster)  [unwired: 1 out]
                        n396 = property class="Instr"(reference=w570, error in=w571) -> (reference out=w575:refnum<visa-resource-name>, error out=w574:errorcluster, "Serial Settings:Number of Bytes at Serial Port"=w573:u32)
                        n397 = VISA Read(VISA resource name=w575, byte count=w573, error in (no error)=w574) -> (VISA resource name out=w577:refnum<visa-resource-name>, error out=w576:errorcluster)  [unwired: 2 out]
                        n398 = VISA Close(VISA resource name=w577, error in (no error)=w576) -> ()  [unwired: 1 out]
                      }
                      frame #1 {
                        n399 = local read "Port for ED33"() -> (w583:refnum<visa-resource-name>)
                        n400 = call-poly "VISA Configure Serial Port"("VISA resource name"=w583, "baud rate (9600)"=u32 115200) -> ("VISA resource name out"=w584:refnum<visa-resource-name>, "error out"=w585:errorcluster)  [unwired: 7 in, 5 out]
                        n401 = flat-sequence {
                          tunnel: w587 -> [w597]
                          tunnel: [w597] -> w588
                          tunnel: [w596] -> w589
                          tunnel: w590 -> [w596]
                          frame #0 {
                            n402 = Wait (ms)(milliseconds to wait=u32 100) -> ()  [unwired: 1 out]
                          }
                        }
                        n403 = VISA Write(VISA resource name=w584, write buffer="write ED33 2", error in (no error)=w585) -> (VISA resource name out=w587:refnum<visa-resource-name>, error out=w590:errorcluster)  [unwired: 1 out]
                        n404 = property class="Instr"(reference=w588, error in=w589) -> (reference out=w593:refnum<visa-resource-name>, error out=w592:errorcluster, "Serial Settings:Number of Bytes at Serial Port"=w591:u32)
                        n405 = VISA Read(VISA resource name=w593, byte count=w591, error in (no error)=w592) -> (VISA resource name out=w595:refnum<visa-resource-name>, error out=w594:errorcluster)  [unwired: 2 out]
                        n406 = VISA Close(VISA resource name=w595, error in (no error)=w594) -> ()  [unwired: 1 out]
                      }
                    }
                    n407 = stacked-sequence {
                      frame #0 {
                        n408 = local read "Port for Sensors"() -> (w551:refnum<visa-resource-name>)
                        n409 = call-poly "VISA Configure Serial Port"("VISA resource name"=w551, "baud rate (9600)"=u32 115200) -> ("VISA resource name out"=w552:refnum<visa-resource-name>, "error out"=w553:errorcluster)  [unwired: 7 in, 5 out]
                        n410 = flat-sequence {
                          tunnel: w554 -> [w564]
                          tunnel: [w564] -> w555
                          tunnel: [w563] -> w556
                          tunnel: w557 -> [w563]
                          frame #0 {
                            n411 = Wait (ms)(milliseconds to wait=u32 100) -> ()  [unwired: 1 out]
                          }
                        }
                        n412 = Concatenate Strings("write buffer", "\n") -> (w548:string)
                        n413 = VISA Write(VISA resource name=w552, write buffer=w548, error in (no error)=w553) -> (VISA resource name out=w554:refnum<visa-resource-name>, error out=w557:errorcluster)  [unwired: 1 out]
                        n414 = property class="Instr"(reference=w555, error in=w556) -> (reference out=w560:refnum<visa-resource-name>, error out=w559:errorcluster, "Serial Settings:Number of Bytes at Serial Port"=w558:u32)
                        n415 = VISA Read(VISA resource name=w560, byte count=w558, error in (no error)=w559) -> (VISA resource name out=w562:refnum<visa-resource-name>, read buffer=→"read buffer":string, error out=w561:errorcluster)  [unwired: 1 out]
                        n416 = VISA Close(VISA resource name=w562, error in (no error)=w561) -> ()  [unwired: 1 out]
                      }
                    }
                    n417 = local write "Operation Done"("Initialised the KOSY3 and sensor stage" ("Operation Done")) -> ()
                    n418 = local write "Current Status"("Home position (0,0,0)" ("Status")) -> ()
                  }
                }
              }
              frame "Import Cordinates" {
                n419 = flat-sequence {
                  frame #0 {
                    n420 = local read "File Path"() -> (w612:path)
                    n421 = call "Dekoder Batch Speicher.vi"("Batchfeld Speicher"=w612) -> ("P9"=w602:dbl[], "P10"=w603:dbl[], "P1"=w604:dbl[], "P2"=w605:dbl[], "P8"=w606:dbl[], "P3"=w607:dbl[], "P4"=w608:dbl[], "P7"=w611:dbl[], "P6"=w609:dbl[], "P5"=w610:dbl[])  [unwired: 5 in]
                    n422 = local write "P9"(w602) -> ()
                    n423 = local write "P10"(w603) -> ()
                    n424 = local write "P1"(w604) -> ()
                    n425 = local write "P2"(w605) -> ()
                    n426 = local write "P8"(w606) -> ()
                    n427 = local write "P3"(w607) -> ()
                    n428 = local write "P4"(w608) -> ()
                    n429 = local write "P5"(w610) -> ()
                    n430 = local write "P6"(w609) -> ()
                    n431 = local write "P7"(w611) -> ()
                  }
                  frame #1 {
                    n432 = local write "Import"(FALSE ("Import")) -> ()
                    n433 = local write "Operation Done"("Import the position cordinates" ("Operation Done")) -> ()
                  }
                }
              }
              frame "Load Sequence" {
                n434 = flat-sequence {
                  frame #0 {
                    n435 = local read "File  Select"() -> (w619:path)
                    n436 = call-poly <vilib>:"Read From Spreadsheet File.vi"("file path (dialog if empty)"=w619) -> ("all rows"=w618:string[][])  [unwired: 6 in, 4 out]
                    n437 = local write "Sequence"(w618) -> ()
                  }
                  frame #1 {
                    n438 = local write "Load Sequence"(FALSE ("Load Sequence")) -> ()
                    n439 = local write "Operation Done"("Sequence loaded" ("Status")) -> ()
                  }
                }
              }
              frame "Manual Control" {
                n440 = flat-sequence {
                  tunnel: [w644] -> w634
                  tunnel: w633 -> [w644]
                  tunnel: [w643] -> w631
                  tunnel: w630 -> [w643]
                  tunnel: [w652] -> w641
                  tunnel: [w651] -> w640
                  tunnel: [w650] -> w639
                  tunnel: [w649] -> w638
                  tunnel: [w648] -> w635
                  tunnel: w634 -> [w648]
                  tunnel: [w647] -> w632
                  tunnel: w631 -> [w647]
                  tunnel: w641 -> [w663]
                  tunnel: w640 -> [w662]
                  tunnel: w639 -> [w661]
                  tunnel: w638 -> [w655]
                  tunnel: [w660] -> w637
                  tunnel: w635 -> [w659]
                  tunnel: w632 -> [w658]
                  tunnel: [w657] -> w627
                  tunnel: [w656] -> w624
                  tunnel: w637 -> [w667]
                  tunnel: [w665] -> w628
                  tunnel: w627 -> [w665]
                  tunnel: [w664] -> w625
                  tunnel: w624 -> [w664]
                  tunnel: cluster{u16, u16, dbl, bool} {36, 1, 0.0, TRUE} -> [w668]
                  tunnel: [w670] -> w629
                  tunnel: w628 -> [w670]
                  tunnel: [w669] -> w626
                  tunnel: w625 -> [w669]
                  tunnel: [w672] -> w623
                  tunnel: w629 -> [w672]
                  tunnel: [w671] -> w622
                  tunnel: w626 -> [w671]
                  frame #0 {
                    w646 = TRUE ("Moving")
                    n441 = Not(x=w646) -> (.not. x?=w645:bool)
                    n442 = local write "Moving"(w646) -> ()
                    n443 = local write "Stopped"(w645) -> ()
                  }
                  frame #1 {
                    n444 = local read "Movement"() -> (w653:T5)
                    n445 = Unbundle(w653) -> ("Axis"=w651:u8, "Direction(To/From)"=w649:u8, "Speed in mm/s\n (5)[0,025-20]"=w650:sgl, "IV6"=w652:bool)
                  }
                  frame #2 {
                    n446 = call <userlib>:"SubVI_Einzelschritte_IF5_IF6.vi"("VISA resource name in"=w659, "Achsen-Wahl (X)"=w662, "Geschwindigkeit\nin mm/s (5)[0,025-20]"=w661, "IF5=F/IF6=T\n(IF6=T) in"=w663, "Schritte oder mm (mm)"="Schritte oder mm (mm)", "error in"=w658, "Richtung (vEw)"=w655) -> ("VISA resource name out"=w657:refnum<visa-resource-name>, "Koordinaten IF6"=w660:T9, "error out"=w656:errorcluster)  [unwired: 2 in, 4 out]
                  }
                  frame #3 {
                    n447 = local write "Current Cordinates"(w667) -> ()
                    n448 = Wait (ms)(milliseconds to wait=100) -> ()  [unwired: 1 out]
                  }
                  frame #4 {
                    n449 = local write "Movement"(w668) -> ()
                  }
                  frame #5 {
                    w675 = FALSE ("Moving")
                    n450 = Not(x=w675) -> (.not. x?=w674:bool)
                    n451 = local write "Moving"(w675) -> ()
                    n452 = local write "Stopped"(w674) -> ()
                    n453 = local write "Operation Done"("Manual movement done" ("Operation Done")) -> ()
                  }
                }
              }
              frame "Move & Measure" {
                n454 = local read "Sensors Active?"() -> (w678:bool)
                n455 = local read "ED33 Active?"() -> (w679:bool)
                n456 = Or(x=w679, y=w678) -> (x .or. y?=w680:bool)
                n457 = case shown="True" w680 {
                  tunnel: w681 -> [_ w688]
                  tunnel: w677 -> [w683 w687]
                  tunnel: [w683 w686] -> w676
                  frame False {
                  }
                  frame True {
                    n458 = flat-sequence {
                      tunnel: w688 -> [w692]
                      tunnel: w687 -> [w690]
                      tunnel: [w689] -> w685
                      tunnel: w685 -> [w947]
                      tunnel: [w947] -> w684
                      tunnel: [w953] -> w686
                      tunnel: w684 -> [w953]
                      frame #0 {
                        n459 = local read "Count"() -> (w691:dbl)
                        n460 = for {
                          N: w691 -> [_]
                          tunnel: w692 -> [w693]
                          tunnel: [w696] -> w689
                          tunnel: w690 -> [w695]
                          n461 = local read "Stop Program"() -> (w694:bool)
                          n462 = case shown="False" w694 {
                            tunnel: w693 -> [w703 _]
                            tunnel: [w700 w936] -> w696
                            tunnel: w695 -> [w698 w936]
                            frame False {
                              w701 = TRUE
                              n463 = local read "Activate Sequence?"() -> (w697:bool)
                              n464 = case shown="True" w697 {
                                tunnel: w703 -> [w707 _]
                                tunnel: [w706 w821] -> w700
                                tunnel: w698 -> [w705 w820]
                                frame False {
                                n465 = case shown="\"PI\", Default" "Y_Axis_Select" {
                                tunnel: w707 -> [w709 w772]
                                tunnel: [w708 w771] -> w706
                                tunnel: w705 -> [w710 w770]
                                frame "PI", Default {
                                n466 = flat-sequence {
                                tunnel: w709 -> [w719]
                                tunnel: [w718] -> w711
                                tunnel: w710 -> [w718]
                                tunnel: [w769] -> w708
                                tunnel: w711 -> [w769]
                                frame #0 {
                                n467 = flat-sequence {
                                tunnel: [w727] -> w722
                                tunnel: [w726] -> w721
                                tunnel: [w725] -> w720
                                tunnel: w719 -> [w723]
                                tunnel: w722 -> [w730]
                                tunnel: w721 -> [w728]
                                tunnel: w720 -> [w733]
                                tunnel: [w731] -> w717
                                tunnel: [w728] -> w715
                                tunnel: [w730] -> w713
                                tunnel: w717 -> [w739]
                                tunnel: [w738] -> w716
                                tunnel: w715 -> [w737]
                                tunnel: [w737] -> w714
                                tunnel: w713 -> [w736]
                                tunnel: [w736] -> w712
                                tunnel: [w745] -> _
                                tunnel: w716 -> [w743]
                                tunnel: w714 -> [w742]
                                tunnel: w712 -> [w741]
                                frame #0 {
                                w726 = 1 ("System no.")
                                n468 = local read "Axes to move Y"() -> (w727:string[])
                                n469 = call "VEL.vi"("System no."=w726, "Axes to set"=w727, "Velocity values"=dbl[] [1.0], "error in"=w723) -> ("error out"=w725:errorcluster)  [unwired: 14 in, 1 out]
                                }
                                frame #1 {
                                n470 = local read "Steps to move-Y"() -> (w729:dbl[])
                                n471 = local write "Moving"(TRUE ("Moving")) -> ()
                                n472 = call "MVR.vi"("System no."=w728, "Axes to move"=w730, "Position values"=w729, "No.of digits"=i16 4, "error in"=w733) -> ("error out"=w731:errorcluster)  [unwired: 14 in]
                                }
                                frame #2 {
                                n473 = call "General wait for movement to stop.vi"("System no."=w737, "Axes to wait for"=w736, "Additional wait time, ms"=u32 500, "error in"=w739) -> ("Stopped"=w735:bool, "error out"=w738:errorcluster)  [unwired: 14 in]
                                n474 = local write "Stopped"(w735) -> ()
                                }
                                frame #3 {
                                n475 = call "POS?.vi"("System no."=w742, "Axes to query"=w741, "error in"=w743) -> ("Position"=w747:dbl[], "error out"=w745:errorcluster)  [unwired: 15 in]
                                n476 = local write "Move Rel Y"(FALSE ("Move Rel")) -> ()
                                n477 = local write "Moving"(FALSE ("Moving")) -> ()
                                n478 = local write "Yaxis Stage"(w747) -> ()
                                }
                                }
                                }
                                frame #1 {
                                n479 = local read "Port for Sensors"() -> (w768:refnum<visa-resource-name>)
                                n480 = local read "Sensors Active?"() -> (w748:bool)
                                n481 = local read "Port for ED33"() -> (w752:refnum<visa-resource-name>)
                                n482 = local read "ED33 Active?"() -> (w749:bool)
                                n483 = local read "Sensor Box"() -> (w750:string)
                                n484 = call "Sensor_Read.vi"("Clear"=FALSE ("ED33 Active?"), "Sensor Box"=w750, "Port Sensors"=w768, "Sensors Active?"=w748, "ED33 Active?"=w749, "Port ED33"=w752) -> ("Sensors_output"=w761:string[][], "ED33_output"=w751:string[][])  [unwired: 4 in]
                                n485 = local write "Sensor_output"(w761) -> ()
                                n486 = local write "ED33_output"(w751) -> ()
                                n487 = Index Array(array=w751, index (col)=1) -> (element=w756:string[])  [unwired: 1 in]
                                n488 = Index Array(array=w761, index (col)=0) -> (element=w765:string[])  [unwired: 1 in]
                                n489 = Index Array(array=w761, index (col)=1) -> (element=w763:string[])  [unwired: 1 in]
                                n490 = Index Array(array=w765) -> (element=w764:string)  [unwired: 1 in]
                                n491 = Index Array(array=w763) -> (element=w762:string)  [unwired: 1 in]
                                n492 = Decimal String To Number(string=w756, default (0L)=i64 0) -> (number=w753:i64[])  [unwired: 1 in, 1 out]
                                n493 = Decimal String To Number(string=w764) -> (number=w760:i32)  [unwired: 2 in, 1 out]
                                n494 = Decimal String To Number(string=w762) -> (number=w759:i32)  [unwired: 2 in, 1 out]
                                n495 = local write "ED33"(w753) -> ()
                                n496 = Bundle(w760, w759) -> (w758:cluster{i32, i32})  [unwired: 1 in]
                                n497 = local write "Sensor"(w758) -> ()
                                }
                                }
                                }
                                frame "KOSY3" {
                                n498 = flat-sequence {
                                tunnel: w772 -> [w781]
                                tunnel: [w780] -> w774
                                tunnel: [w779] -> w773
                                tunnel: w770 -> [w777]
                                tunnel: w774 -> [w818]
                                tunnel: [w819] -> w771
                                tunnel: w773 -> [w819]
                                frame #0 {
                                n499 = local read "X axis"() -> (w787:enum16{"Left", "Right"})
                                n500 = case shown="\"Right\"" w787 {
                                tunnel: [1 0] -> w790
                                frame "Left", Default {
                                }
                                frame "Right" {
                                }
                                }
                                n501 = local read "Y axis"() -> (w785:enum16{"Forward", "Backward"})
                                n502 = case shown="\"Forward\", Default" w785 {
                                tunnel: [0 1] -> w789
                                frame "Forward", Default {
                                }
                                frame "Backward" {
                                }
                                }
                                n503 = local read "Z axis"() -> (w786:enum16{"Up", "Down"})
                                n504 = case shown="\"Down\"" w786 {
                                tunnel: [1 0] -> w788
                                frame "Up", Default {
                                }
                                frame "Down" {
                                }
                                }
                                n505 = local read "Steps(mm)"() -> (w778:dbl[])
                                n506 = local read "Activate Sequence?"() -> (w784:bool)
                                n507 = local read "Current Sequence"() -> (w783:string[])
                                n508 = Build Array (concatenate)(w778, w790, w789, w788) -> (w775:dbl[])
                                n509 = call "Go Straight.vi"("VISA resource name in"=w777, "Sequence Active"=w784, "Current sequence"=w783, "Speed"=1.0, "Steps(mm)"=w775, "error in"=w781) -> ("VISA resource name out"=w779:refnum<visa-resource-name>, "Koordinaten IF6"=w782:T9, "error out"=w780:errorcluster)
                                n510 = local write "Current Cordinates"(w782) -> ()
                                }
                                frame #1 {
                                n511 = local read "Port for Sensors"() -> (w817:refnum<visa-resource-name>)
                                n512 = local read "Sensors Active?"() -> (w797:bool)
                                n513 = local read "Port for ED33"() -> (w801:refnum<visa-resource-name>)
                                n514 = local read "ED33 Active?"() -> (w798:bool)
                                n515 = local read "Sensor Box"() -> (w799:string)
                                n516 = call "Sensor_Read.vi"("error in (no error)"=w818, "Clear"=FALSE ("ED33 Active?"), "Sensor Box"=w799, "Port Sensors"=w817, "Sensors Active?"=w797, "ED33 Active?"=w798, "Port ED33"=w801) -> ("Sensors_output"=w810:string[][], "ED33_output"=w800:string[][])  [unwired: 3 in]
                                n517 = local write "Sensor_output"(w810) -> ()
                                n518 = local write "ED33_output"(w800) -> ()
                                n519 = Index Array(array=w800, index (col)=1) -> (element=w805:string[])  [unwired: 1 in]
                                n520 = Index Array(array=w810, index (col)=0) -> (element=w814:string[])  [unwired: 1 in]
                                n521 = Index Array(array=w810, index (col)=1) -> (element=w812:string[])  [unwired: 1 in]
                                n522 = Index Array(array=w814) -> (element=w813:string)  [unwired: 1 in]
                                n523 = Index Array(array=w812) -> (element=w811:string)  [unwired: 1 in]
                                n524 = Decimal String To Number(string=w805, default (0L)=i64 0) -> (number=w802:i64[])  [unwired: 1 in, 1 out]
                                n525 = Decimal String To Number(string=w813) -> (number=w809:i32)  [unwired: 2 in, 1 out]
                                n526 = Decimal String To Number(string=w811) -> (number=w808:i32)  [unwired: 2 in, 1 out]
                                n527 = local write "ED33"(w802) -> ()
                                n528 = Bundle(w809, w808) -> (w807:cluster{i32, i32})  [unwired: 1 in]
                                n529 = local write "Sensor"(w807) -> ()
                                }
                                }
                                }
                                }
                                }
                                frame True {
                                n530 = local read "Current Sequence"() -> (w824:string[])
                                n531 = Index Array(array=w824, index=1) -> (element=w822:string)
                                n532 = case shown="\"PI\", Default" w822 {
                                tunnel: [w827 w890] -> w821
                                tunnel: w820 -> [w825 _]
                                frame "PI", Default {
                                n533 = flat-sequence {
                                tunnel: [w828] -> w826
                                tunnel: w825 -> [w828]
                                tunnel: [w868] -> w827
                                tunnel: w826 -> [w868]
                                frame #0 {
                                n534 = flat-sequence {
                                tunnel: [w841] -> w837
                                tunnel: [w840] -> w836
                                tunnel: [w839] -> w835
                                tunnel: w837 -> [w849]
                                tunnel: w836 -> [w848]
                                tunnel: w835 -> [w852]
                                tunnel: [w850] -> w834
                                tunnel: [w848] -> w832
                                tunnel: [w849] -> w830
                                tunnel: w834 -> [w858]
                                tunnel: [w857] -> w833
                                tunnel: w832 -> [w856]
                                tunnel: [w856] -> w831
                                tunnel: w830 -> [w855]
                                tunnel: [w855] -> w829
                                tunnel: [w864] -> _
                                tunnel: w833 -> [w862]
                                tunnel: w831 -> [w861]
                                tunnel: w829 -> [w860]
                                frame #0 {
                                w840 = 1 ("System no.")
                                n535 = local read "Axes to move Y"() -> (w841:string[])
                                n536 = call "VEL.vi"("System no."=w840, "Axes to set"=w841, "Velocity values"=dbl[] [2.0]) -> ("error out"=w839:errorcluster)  [unwired: 15 in, 1 out]
                                }
                                frame #1 {
                                w844 = 0.0 ("element")
                                n537 = local read "Current Sequence"() -> (w846:string[])
                                n538 = local write "Moving"(TRUE ("Moving")) -> ()
                                n539 = Index Array(array=w846, index=2) -> (element=w845:string)
                                n540 = Fract/Exp String To Number(string=w845) -> (number=w843:dbl)  [unwired: 3 in, 1 out]
                                n541 = Build Array(w843, w844, w844, w844) -> (w842:dbl[])
                                n542 = call "MVR.vi"("System no."=w848, "Axes to move"=w849, "Position values"=w842, "No.of digits"=i16 4, "error in"=w852) -> ("error out"=w850:errorcluster)  [unwired: 14 in]
                                }
                                frame #2 {
                                n543 = call "General wait for movement to stop.vi"("System no."=w856, "Axes to wait for"=w855, "Additional wait time, ms"=u32 500, "error in"=w858) -> ("Stopped"=w854:bool, "error out"=w857:errorcluster)  [unwired: 14 in]
                                n544 = local write "Stopped"(w854) -> ()
                                }
                                frame #3 {
                                n545 = call "POS?.vi"("System no."=w861, "Axes to query"=w860, "error in"=w862) -> ("Position"=w866:dbl[], "error out"=w864:errorcluster)  [unwired: 15 in]
                                n546 = local write "Move Rel Y"(FALSE ("Move Rel")) -> ()
                                n547 = local write "Moving"(FALSE ("Moving")) -> ()
                                n548 = local write "Yaxis Stage"(w866) -> ()
                                }
                                }
                                }
                                frame #1 {
                                n549 = local read "Port for Sensors"() -> (w889:refnum<visa-resource-name>)
                                n550 = local read "Sensors Active?"() -> (w869:bool)
                                n551 = local read "Port for ED33"() -> (w873:refnum<visa-resource-name>)
                                n552 = local read "ED33 Active?"() -> (w870:bool)
                                n553 = local read "Sensor Box"() -> (w871:string)
                                n554 = call "Sensor_Read.vi"("Clear"=FALSE ("ED33 Active?"), "Sensor Box"=w871, "Port Sensors"=w889, "Sensors Active?"=w869, "ED33 Active?"=w870, "Port ED33"=w873) -> ("Sensors_output"=w882:string[][], "ED33_output"=w872:string[][])  [unwired: 4 in]
                                n555 = local write "Sensor_output"(w882) -> ()
                                n556 = local write "ED33_output"(w872) -> ()
                                n557 = Index Array(array=w872, index (col)=1) -> (element=w877:string[])  [unwired: 1 in]
                                n558 = Index Array(array=w882, index (col)=0) -> (element=w886:string[])  [unwired: 1 in]
                                n559 = Index Array(array=w882, index (col)=1) -> (element=w884:string[])  [unwired: 1 in]
                                n560 = Index Array(array=w886) -> (element=w885:string)  [unwired: 1 in]
                                n561 = Index Array(array=w884) -> (element=w883:string)  [unwired: 1 in]
                                n562 = Decimal String To Number(string=w877, default (0L)=i64 0) -> (number=w874:i64[])  [unwired: 1 in, 1 out]
                                n563 = Decimal String To Number(string=w885) -> (number=w881:i32)  [unwired: 2 in, 1 out]
                                n564 = Decimal String To Number(string=w883) -> (number=w880:i32)  [unwired: 2 in, 1 out]
                                n565 = local write "ED33"(w874) -> ()
                                n566 = Get Date/Time In Seconds() -> (seconds since 1Jan1904=→"current time":timestamp)
                                n567 = Bundle(w881, w880) -> (w879:cluster{i32, i32})  [unwired: 1 in]
                                n568 = local write "Sensor"(w879) -> ()
                                }
                                }
                                }
                                frame "KOSY3" {
                                n569 = flat-sequence {
                                tunnel: [w897] -> w892
                                tunnel: [w896] -> w891
                                tunnel: w892 -> [w934]
                                tunnel: [w935] -> w890
                                tunnel: w891 -> [w935]
                                frame #0 {
                                n570 = local read "X axis"() -> (w903:enum16{"Left", "Right"})
                                n571 = case shown="\"Right\"" w903 {
                                tunnel: [1 0] -> w906
                                frame "Left", Default {
                                }
                                frame "Right" {
                                }
                                }
                                n572 = local read "Y axis"() -> (w901:enum16{"Forward", "Backward"})
                                n573 = case shown="\"Forward\", Default" w901 {
                                tunnel: [0 1] -> w905
                                frame "Forward", Default {
                                }
                                frame "Backward" {
                                }
                                }
                                n574 = local read "Z axis"() -> (w902:enum16{"Up", "Down"})
                                n575 = case shown="\"Down\"" w902 {
                                tunnel: [1 0] -> w904
                                frame "Up", Default {
                                }
                                frame "Down" {
                                }
                                }
                                n576 = local read "Steps(mm)"() -> (w895:dbl[])
                                n577 = local read "Activate Sequence?"() -> (w900:bool)
                                n578 = local read "Current Sequence"() -> (w899:string[])
                                n579 = Build Array (concatenate)(w895, w906, w905, w904) -> (w893:dbl[])
                                n580 = call "Go Straight.vi"("Sequence Active"=w900, "Current sequence"=w899, "Speed"=1.0, "Steps(mm)"=w893) -> ("VISA resource name out"=w896:refnum<visa-resource-name>, "Koordinaten IF6"=w898:T9, "error out"=w897:errorcluster)  [unwired: 2 in]
                                n581 = local write "Current Cordinates"(w898) -> ()
                                }
                                frame #1 {
                                n582 = local read "Port for Sensors"() -> (w933:refnum<visa-resource-name>)
                                n583 = local read "Sensors Active?"() -> (w913:bool)
                                n584 = local read "Port for ED33"() -> (w917:refnum<visa-resource-name>)
                                n585 = local read "ED33 Active?"() -> (w914:bool)
                                n586 = local read "Sensor Box"() -> (w915:string)
                                n587 = call "Sensor_Read.vi"("error in (no error)"=w934, "Clear"=FALSE ("ED33 Active?"), "Sensor Box"=w915, "Port Sensors"=w933, "Sensors Active?"=w913, "ED33 Active?"=w914, "Port ED33"=w917) -> ("Sensors_output"=w926:string[][], "ED33_output"=w916:string[][])  [unwired: 3 in]
                                n588 = local write "Sensor_output"(w926) -> ()
                                n589 = local write "ED33_output"(w916) -> ()
                                n590 = Index Array(array=w916, index (col)=1) -> (element=w921:string[])  [unwired: 1 in]
                                n591 = Index Array(array=w926, index (col)=0) -> (element=w930:string[])  [unwired: 1 in]
                                n592 = Index Array(array=w926, index (col)=1) -> (element=w928:string[])  [unwired: 1 in]
                                n593 = Index Array(array=w930) -> (element=w929:string)  [unwired: 1 in]
                                n594 = Index Array(array=w928) -> (element=w927:string)  [unwired: 1 in]
                                n595 = Decimal String To Number(string=w921, default (0L)=i64 0) -> (number=w918:i64[])  [unwired: 1 in, 1 out]
                                n596 = Decimal String To Number(string=w929) -> (number=w925:i32)  [unwired: 2 in, 1 out]
                                n597 = Decimal String To Number(string=w927) -> (number=w924:i32)  [unwired: 2 in, 1 out]
                                n598 = local write "ED33"(w918) -> ()
                                n599 = Bundle(w925, w924) -> (w923:cluster{i32, i32})  [unwired: 1 in]
                                n600 = local write "Sensor"(w923) -> ()
                                }
                                }
                                }
                                }
                                }
                              }
                              n601 = Not(x=w701) -> (.not. x?=w702:bool)
                              n602 = local write "Moving"(w701) -> ()
                              n603 = local write "Stopped"(w702) -> ()
                              n604 = local write "Current Status"("Move and measure") -> ()
                            }
                            frame True {
                            }
                          }
                        }
                      }
                      frame #1 {
                        n605 = local read "Steps(mm)"() -> (w937:dbl[])
                        n606 = local read "Current Cordinates"() -> (w942:T7)
                        n607 = local read "Sensors Active?"() -> (w944:bool)
                        n608 = local read "Sensor_output"() -> (w941:string[][])
                        n609 = local read "ED33 Active?"() -> (w940:bool)
                        n610 = local read "ED33_output"() -> (w939:string[][])
                        n611 = local read "Sensor Box"() -> (w946:string)
                        n612 = Index Array(array=w937, index=1) -> (element=w943:dbl)
                        n613 = call "Sensor_Save.vi"("ED33_output"=w939, "Sensor_output"=w941, "ED33 Active?"=w940, "Current Cordinates"=w942, "Sensor Box"=w946, "Cont/MM"="Move&Measure" ("Movement"), "Sensors Active?"=w944, "Min_move"=w943) -> ()
                      }
                      frame #2 {
                        w948 = TRUE
                        w952 = FALSE
                        n614 = local write "Clear Sensor Readings"(TRUE ("Clear Sensor Readings")) -> ()
                        n615 = Not(x=w948) -> (.not. x?=w949:bool)
                        n616 = local write "Stopped"(w948) -> ()
                        n617 = local write "Sensors Active?"(w952) -> ()
                        n618 = local write "ED33 Active?"(w952) -> ()
                        n619 = local write "Move & Measure"(w952) -> ()
                        n620 = local write "Moving"(w949) -> ()
                        n621 = local write "Operation Done"("Moved and Measured") -> ()
                      }
                    }
                  }
                }
              }
              frame "Move WithRef" {
                n622 = flat-sequence {
                  tunnel: w959 -> [w964]
                  tunnel: w962 -> [w965]
                  tunnel: [w965] -> w955
                  tunnel: [w964] -> w954
                  tunnel: [w967] -> w961
                  tunnel: [w972] -> w958
                  tunnel: w955 -> [w967]
                  tunnel: w954 -> [w972]
                  tunnel: w961 -> [w976]
                  tunnel: [w980] -> w960
                  tunnel: w958 -> [w979]
                  tunnel: [w978] -> w957
                  frame #0 {
                    w963 = i64 0 ("ED33_pos")
                    n623 = local write "ED33_pos"(w963) -> ()
                    n624 = local write "Ref_Steps"(w963) -> ()
                    n625 = local write "Diff"(w963) -> ()
                  }
                  frame #1 {
                    n626 = local read "Port for ED33"() -> (w973:refnum<visa-resource-name>)
                    n627 = call "Sensor_Read.vi"("ED33 Active?"=TRUE, "Port ED33"=w973) -> ("ED33_output"=w974:string[][])  [unwired: 8 in, 1 out]
                    n628 = Index Array(array=w974, index (col)=0 ("disabled index (col)")) -> (element=w966:string[])  [unwired: 1 in]
                    n629 = local write "Sensor Output"(w966) -> ()
                    n630 = Index Array(array=w966) -> (element=w970:string)  [unwired: 1 in]
                    n631 = Scan Value(string=w970, format string="") -> (value=w968:dbl)  [unwired: 1 in, 1 out]
                    n632 = local write "ED33_pos"(w968) -> ()
                    n633 = local write "Ref_Steps"(w968) -> ()
                  }
                  frame #2 {
                    n634 = case shown="\"5mm\", Default" "Pole Pitch" {
                      tunnel: w976 -> [w988 w1082]
                      tunnel: [w987 w1081] -> w980
                      tunnel: w979 -> [w986 w1080]
                      tunnel: [w985 w1079] -> w978
                      frame "5mm", Default {
                        n635 = flat-sequence {
                          tunnel: w988 -> [w999]
                          tunnel: [w992] -> w984
                          tunnel: w986 -> [w991]
                          tunnel: [w990] -> w983
                          tunnel: w984 -> [w1017]
                          tunnel: w983 -> [w1015]
                          tunnel: [w1016] -> w982
                          tunnel: [w1014] -> w981
                          tunnel: [w1059] -> w985
                          tunnel: [w1061] -> w987
                          tunnel: w982 -> [w1062]
                          tunnel: w981 -> [w1060]
                          frame #0 {
                            n636 = local read "X axis"() -> (w1002:enum16{"Left", "Right"})
                            n637 = local read "Y axis"() -> (w1001:enum16{"Forward", "Backward"})
                            n638 = local read "Z axis"() -> (w1000:enum16{"Up", "Down"})
                            n639 = case shown="\"Left\", Default" w1002 {
                              tunnel: [1 0] -> w1006
                              frame "Left", Default {
                              }
                              frame "Right" {
                              }
                            }
                            n640 = case shown="\"Forward\", Default" w1001 {
                              tunnel: [0 1] -> w1005
                              frame "Forward", Default {
                              }
                              frame "Backward" {
                              }
                            }
                            n641 = case shown="\"Up\", Default" w1000 {
                              tunnel: [1 0] -> w1004
                              frame "Up", Default {
                              }
                              frame "Down" {
                              }
                            }
                            n642 = Build Array(0.0, 4.9, 0.0) -> (w993:dbl[])
                            n643 = Build Array (concatenate)(w993, w1006, w1005, w1004) -> (w997:dbl[])
                            n644 = call "Go Straight.vi"("VISA resource name in"=w999, "Sequence Active"=FALSE, "Speed"=3.0, "Steps(mm)"=w997, "error in"=w991) -> ("VISA resource name out"=w992:refnum<visa-resource-name>, "Koordinaten IF6"=w998:T9, "error out"=w990:errorcluster)  [unwired: 1 in]
                            n645 = local write "Current Cordinates"(w998) -> ()
                          }
                          frame #1 {
                            n646 = for {
                              N: 8 -> [_]
                              tunnel: w1017 -> [w1023]
                              tunnel: [w1021] -> w1016
                              tunnel: w1015 -> [w1020]
                              tunnel: [w1019] -> w1014
                              n647 = flat-sequence {
                                tunnel: w1023 -> [w1029]
                                tunnel: [w1027] -> w1022
                                tunnel: w1020 -> [w1026]
                                tunnel: [w1025] -> w1018
                                tunnel: w1022 -> [w1034]
                                tunnel: [w1034] -> w1021
                                tunnel: [w1032] -> w1019
                                tunnel: w1018 -> [w1032]
                                frame #0 {
                                n648 = local read "Activate Sequence?"() -> (w1024:bool)
                                n649 = local read "Current Sequence"() -> (w1030:string[])
                                n650 = call "Go Straight.vi"("VISA resource name in"=w1029, "Sequence Active"=w1024, "Current sequence"=w1030, "Speed"=1.0, "error in"=w1026) -> ("VISA resource name out"=w1027:refnum<visa-resource-name>, "Koordinaten IF6"=w1028:T9, "error out"=w1025:errorcluster)  [unwired: 1 in]
                                n651 = local write "Current Cordinates"(w1028) -> ()
                                }
                                frame #1 {
                                n652 = local read "Port for ED33"() -> (w1033:refnum<visa-resource-name>)
                                n653 = call "Sensor_Read.vi"("ED33 Active?"=TRUE, "Port ED33"=w1033) -> ("ED33_output"=w1043:string[][])  [unwired: 8 in, 1 out]
                                n654 = Index Array(array=w1043, index (col)=0 ("disabled index (col)")) -> (element=w1041:string[])  [unwired: 1 in]
                                n655 = Index Array(array=w1041) -> (element=w1038:string)  [unwired: 1 in]
                                n656 = local read "Ref_Steps"() -> (w1036:i64)
                                n657 = Scan Value(string=w1038, format string="") -> (value=w1037:dbl)  [unwired: 1 in, 1 out]
                                n658 = Subtract(x=w1036, y=w1037) -> (x-y=w1035:dbl)
                                n659 = local write "ED33_pos"(w1037) -> ()
                                n660 = local write "Diff"(w1035) -> ()
                                }
                              }
                            }
                          }
                          frame #2 {
                            n661 = local read "Diff"() -> (w1056:i64)
                            n662 = Subtract(x=i64 1000000, y=w1056) -> (x-y=w1071:i64)
                            n663 = Multiply(x=w1071, y=0.005) -> (x*y=w1070:dbl)
                            n664 = Divide(x=w1070, y=1000.0) -> (x/y=w1052:dbl)
                            n665 = local read "X axis"() -> (w1066:enum16{"Left", "Right"})
                            n666 = local read "Y axis"() -> (w1065:enum16{"Forward", "Backward"})
                            n667 = local read "Z axis"() -> (w1064:enum16{"Up", "Down"})
                            n668 = Multiply(x=w1052, y=100.0) -> (x*y=w1055:dbl)
                            n669 = Round To Nearest(number=w1055) -> (nearest integer value=w1054:dbl)
                            n670 = case shown="\"Left\", Default" w1066 {
                              tunnel: [1 0] -> w1048
                              frame "Left", Default {
                              }
                              frame "Right" {
                              }
                            }
                            n671 = case shown="\"Forward\", Default" w1065 {
                              tunnel: [0 1] -> w1049
                              frame "Forward", Default {
                              }
                              frame "Backward" {
                              }
                            }
                            n672 = case shown="\"Up\", Default" w1064 {
                              tunnel: [1 0] -> w1050
                              frame "Up", Default {
                              }
                              frame "Down" {
                              }
                            }
                            n673 = Divide(x=w1054, y=100.0) -> (x/y=w1047:dbl)
                            n674 = Build Array(0.0 ("element"), w1047, 0.0 ("element")) -> (w1044:dbl[])
                            n675 = Build Array (concatenate)(w1044, w1048, w1049, w1050) -> (w1068:dbl[])
                            n676 = call "Go Straight.vi"("VISA resource name in"=w1062, "Sequence Active"=FALSE, "Speed"=0.5, "Steps(mm)"=w1068, "error in"=w1060) -> ("VISA resource name out"=w1061:refnum<visa-resource-name>, "Koordinaten IF6"=w1058:T9, "error out"=w1059:errorcluster)  [unwired: 1 in]
                            n677 = local write "Current Cordinates"(w1058) -> ()
                          }
                        }
                      }
                      frame "1mm" {
                        n678 = while {
                          tunnel: w1082 -> [w1091]
                          tunnel: [w1090] -> w1081
                          tunnel: w1080 -> [w1088]
                          tunnel: [w1086] -> w1079
                          stop <- w1084 stop-if-true
                          n679 = local read "Diff"() -> (w1085:i64)
                          n680 = flat-sequence {
                            tunnel: w1091 -> [w1092]
                            tunnel: [w1095] -> w1089
                            tunnel: w1088 -> [w1094]
                            tunnel: [w1093] -> w1087
                            tunnel: [w1121] -> w1090
                            tunnel: w1089 -> [w1121]
                            tunnel: w1087 -> [w1120]
                            tunnel: [w1120] -> w1086
                            frame #0 {
                              n681 = local read "X axis"() -> (w1097:enum16{"Left", "Right"})
                              n682 = local read "Y axis"() -> (w1098:enum16{"Forward", "Backward"})
                              n683 = local read "Z axis"() -> (w1099:enum16{"Up", "Down"})
                              n684 = case shown="\"Left\", Default" w1097 {
                                tunnel: [1 0] -> w1106
                                frame "Left", Default {
                                }
                                frame "Right" {
                                }
                              }
                              n685 = case shown="\"Forward\", Default" w1098 {
                                tunnel: [0 1] -> w1105
                                frame "Forward", Default {
                                }
                                frame "Backward" {
                                }
                              }
                              n686 = case shown="\"Up\", Default" w1099 {
                                tunnel: [1 0] -> w1104
                                frame "Up", Default {
                                }
                                frame "Down" {
                                }
                              }
                              n687 = local read "Steps(mm)"() -> (w1096:dbl[])
                              n688 = local read "Activate Sequence?"() -> (w1102:bool)
                              n689 = local read "Current Sequence"() -> (w1101:string[])
                              n690 = Build Array (concatenate)(w1096, w1106, w1105, w1104) -> (w1103:dbl[])
                              n691 = call "Go Straight.vi"("VISA resource name in"=w1092, "Sequence Active"=w1102, "Current sequence"=w1101, "Speed"=1.0, "Steps(mm)"=w1103, "error in"=w1094) -> ("VISA resource name out"=w1095:refnum<visa-resource-name>, "Koordinaten IF6"=w1100:T9, "error out"=w1093:errorcluster)
                              n692 = local write "Current Cordinates"(w1100) -> ()
                            }
                            frame #1 {
                              n693 = local read "Port for ED33"() -> (w1123:refnum<visa-resource-name>)
                              n694 = call "Sensor_Read.vi"("ED33 Active?"=TRUE, "Port ED33"=w1123) -> ("ED33_output"=w1125:string[][])  [unwired: 8 in, 1 out]
                              n695 = Index Array(array=w1125, index (col)=0 ("disabled index (col)")) -> (element=w1122:string[])  [unwired: 1 in]
                              n696 = Index Array(array=w1122) -> (element=w1118:string)  [unwired: 1 in]
                              n697 = local read "Ref_Steps"() -> (w1115:i64)
                              n698 = Scan Value(string=w1118, format string="") -> (value=w1114:dbl)  [unwired: 1 in, 1 out]
                              n699 = Subtract(x=w1115, y=w1114) -> (x-y=w1116:dbl)
                              n700 = local write "ED33_pos"(w1114) -> ()
                              n701 = local write "Diff"(w1116) -> ()
                            }
                          }
                          n702 = Greater Or Equal?(x=w1085, y=198000 ("8")) -> (x >= y?=w1084:bool)
                        }
                      }
                    }
                  }
                }
              }
              frame "Reset Position" {
                n703 = flat-sequence {
                  frame #0 {
                    n704 = local read "Position"() -> (w1129:T3)
                    n705 = case shown="\"Position 10\"" w1129 {
                      tunnel: dbl[] [0.0, 0.0, 0.0] ("P1") -> [w1131 w1132 w1133 w1134 w1135 w1136 w1137 w1138 w1139 w1140]
                      frame "Position 1", Default {
                        n706 = local write "P1"(w1131) -> ()
                      }
                      frame "Position 2" {
                        n707 = local write "P2"(w1132) -> ()
                      }
                      frame "Position 3" {
                        n708 = local write "P3"(w1133) -> ()
                      }
                      frame "Position 4" {
                        n709 = local write "P4"(w1134) -> ()
                      }
                      frame "Position 5" {
                        n710 = local write "P5"(w1135) -> ()
                      }
                      frame "Position 6" {
                        n711 = local write "P6"(w1136) -> ()
                      }
                      frame "Position 7" {
                        n712 = local write "P7"(w1137) -> ()
                      }
                      frame "Position 8" {
                        n713 = local write "P8"(w1138) -> ()
                      }
                      frame "Position 9" {
                        n714 = local write "P9"(w1139) -> ()
                      }
                      frame "Position 10" {
                        n715 = local write "P10"(w1140) -> ()
                      }
                    }
                  }
                  frame #1 {
                    n716 = local write "Reset"(FALSE ("Reset")) -> ()
                    n717 = local write "Operation Done"("The selected position is reset" ("Operation Done")) -> ()
                  }
                }
              }
              frame "Reset All" {
                n718 = flat-sequence {
                  frame #0 {
                    w1146 = dbl[] [0.0, 0.0, 0.0] ("P1")
                    n719 = local write "P1"(w1146) -> ()
                    n720 = local write "P2"(w1146) -> ()
                    n721 = local write "P3"(w1146) -> ()
                    n722 = local write "P4"(w1146) -> ()
                    n723 = local write "P5"(w1146) -> ()
                    n724 = local write "P6"(w1146) -> ()
                    n725 = local write "P7"(w1146) -> ()
                    n726 = local write "P8"(w1146) -> ()
                    n727 = local write "P9"(w1146) -> ()
                    n728 = local write "P10"(w1146) -> ()
                    n729 = local write "Steps(mm)"(w1146) -> ()
                  }
                  frame #1 {
                    n730 = local write "Reset All"(FALSE ("Reset all Positions")) -> ()
                    n731 = local write "Operation Done"("Reset all positions" ("Operation Done")) -> ()
                  }
                }
              }
              frame "Read Sensors" {
                n732 = local read "Activate Sequence?"() -> (w1149:bool)
                n733 = case shown="False" w1149 {
                  frame False {
                    n734 = local read "Sensors Active?"() -> (w1153:bool)
                    n735 = local read "ED33 Active?"() -> (w1154:bool)
                    n736 = case shown="True" w1154 {
                      frame True {
                        n737 = flat-sequence {
                          frame #0 {
                            w1167 = FALSE ("Sensors Active?")
                            n738 = local read "Port for ED33"() -> (w1165:refnum<visa-resource-name>)
                            n739 = Not(x=w1167) -> (.not. x?=w1166:bool)
                            n740 = call "Sensor_Read.vi"("Sensors Active?"=w1167, "ED33 Active?"=w1166, "Port ED33"=w1165) -> ("ED33_output"=w1164:string[][])  [unwired: 7 in, 1 out]
                            n741 = Index Array(array=w1164, index (row)=0 ("disabled index (col)")) -> (element=→"Sensor Output":string[])  [unwired: 1 in]
                          }
                          frame #1 {
                            w1168 = FALSE ("Read Sensor")
                            n742 = local write "Read Sensor"(w1168) -> ()
                            n743 = local write "ED33 Active?"(w1168) -> ()
                          }
                        }
                      }
                      frame False {
                      }
                    }
                    n744 = case shown="True" w1153 {
                      frame False {
                      }
                      frame True {
                        n745 = flat-sequence {
                          frame #0 {
                            w1160 = FALSE ("ED33 Active?")
                            n746 = local read "Port for Sensors"() -> (w1158:refnum<visa-resource-name>)
                            n747 = Not(x=w1160) -> (.not. x?=w1159:bool)
                            n748 = call "Sensor_Read.vi"("Port Sensors"=w1158, "Sensors Active?"=w1159, "ED33 Active?"=w1160) -> ("Sensors_output"=w1157:string[][])  [unwired: 7 in, 1 out]
                            n749 = Index Array(array=w1157, index (row)=0) -> (element=w1155:string[])  [unwired: 1 in]
                            n750 = local write "Sensor Output"(w1155) -> ()
                          }
                          frame #1 {
                            w1161 = FALSE ("Read Sensor")
                            n751 = local write "Read Sensor"(w1161) -> ()
                            n752 = local write "Sensors Active?"(w1161) -> ()
                          }
                        }
                      }
                    }
                  }
                  frame True {
                    n753 = flat-sequence {
                      frame #0 {
                        n754 = local read "Current Sequence"() -> (w1171:string[])
                        n755 = Index Array(array=w1171, index=1) -> (element=w1169:string)
                        n756 = case shown="\"ED33\"" w1169 {
                          frame "Sensors", Default {
                            n757 = local read "Current Sequence"() -> (w1173:string[])
                            n758 = local write "Sensors Active?"(TRUE ("ED32i Active?")) -> ()
                            n759 = Index Array(array=w1173, index=2) -> (element=w1172:string)
                            n760 = local write "Sensor Box"(w1172) -> ()
                          }
                          frame "ED33" {
                            n761 = local write "ED33 Active?"(TRUE ("ED33 Active?")) -> ()
                          }
                        }
                      }
                      frame #1 {
                        n762 = local write "Operation Done"("Sensor selected") -> ()
                      }
                    }
                  }
                }
              }
              frame "Save Positions" {
                n763 = flat-sequence {
                  frame #0 {
                    n764 = local read "Current Cordinates"() -> (w1184:T7)
                    n765 = Unbundle(w1184) -> ("X axis"=w1181:sgl, "Y axis"=w1182:sgl, "Z axis"=w1183:sgl)  [unwired: 4 out]
                    n766 = local read "Position"() -> (w1186:T3)
                    n767 = Build Array(w1181, w1182, w1183) -> (w1185:sgl[])
                    n768 = case shown="\"Position 1\", Default" w1186 {
                      tunnel: w1185 -> [w1187 w1188 w1189 w1190 w1191 w1192 w1193 w1194 w1195 w1196]
                      frame "Position 1", Default {
                        n769 = local write "P1"(w1187) -> ()
                      }
                      frame "Position 2" {
                        n770 = local write "P2"(w1188) -> ()
                      }
                      frame "Position 3" {
                        n771 = local write "P3"(w1189) -> ()
                      }
                      frame "Position 4" {
                        n772 = local write "P4"(w1190) -> ()
                      }
                      frame "Position 5" {
                        n773 = local write "P5"(w1191) -> ()
                      }
                      frame "Position 6" {
                        n774 = local write "P6"(w1192) -> ()
                      }
                      frame "Position 7" {
                        n775 = local write "P7"(w1193) -> ()
                      }
                      frame "Position 8" {
                        n776 = local write "P8"(w1194) -> ()
                      }
                      frame "Position 9" {
                        n777 = local write "P9"(w1195) -> ()
                      }
                      frame "Position 10" {
                        n778 = local write "P10"(w1196) -> ()
                      }
                    }
                  }
                  frame #1 {
                    n779 = local write "Save"(FALSE ("Save Button")) -> ()
                    n780 = local write "Operation Done"("Position cordinates saved" ("Operation Done")) -> ()
                  }
                }
              }
              frame "Set Speed" {
                n781 = flat-sequence {
                  frame #0 {
                    n782 = local read "Current Sequence"() -> (w1202:string[])
                    n783 = Index Array(array=w1202, index=1) -> (element=w1204:string)
                    n784 = Fract/Exp String To Number(string=w1204) -> (number=w1205:dbl)  [unwired: 3 in, 1 out]
                    n785 = local write "Speed"(w1205) -> ()
                  }
                  frame #1 {
                    n786 = local write "Operation Done"("Speed Set") -> ()
                  }
                }
              }
              frame "Set Powersupply" {
                n787 = flat-sequence {
                  frame #0 {
                    n788 = local read "Current Sequence"() -> (w1210:string[])
                    n789 = local read "Port for Powersupply"() -> (w1216:refnum<visa-resource-name>)
                    n790 = Index Array(array=w1210, index=1 ("Index")) -> (element=w1212:string)
                    n791 = Concatenate Strings(w1212, "\r") -> (w1214:string)
                    n792 = call "Serial_com_powersupply für Funktion.vi"("VISA resource name"=w1216, "write"=TRUE, "string to write"=w1214) -> ()  [unwired: 6 in, 2 out]
                  }
                  frame #1 {
                    n793 = local read "Port for Write Head"() -> (w1218:refnum<visa-resource-name>)
                    n794 = Concatenate Strings("GPV 6" ("string"), "\r") -> (w1220:string)
                    n795 = call "Serial_com_powersupply für Funktion.vi"("VISA resource name"=w1218, "write"=TRUE, "string to write"=w1220) -> ()  [unwired: 6 in, 2 out]
                  }
                  frame #2 {
                    n796 = local write "Operation Done"("Powersupply Set") -> ()
                  }
                }
              }
              frame "Set PolePitch" {
                n797 = flat-sequence {
                  frame #0 {
                    n798 = local read "Current Sequence"() -> (w1227:string[])
                    n799 = Index Array(array=w1227, index=1) -> (element=w1226:string)
                    n800 = local write "Pole Pitch"(w1226) -> ()
                  }
                  frame #1 {
                    n801 = local write "Operation Done"("Pole pitch set" ("Operation Done")) -> ()
                  }
                }
              }
              frame "Set Steps" {
                n802 = flat-sequence {
                  frame #0 {
                    n803 = for {
                      N: 7 -> [_]
                      tunnel: [w1253] -> w1235 mode=indexing
                      i -> [w1254]
                      n804 = local read "Current Sequence"() -> (w1255:string[])
                      n805 = Increment(x=w1254) -> (x+1=w1257:i32)
                      n806 = Index Array(array=w1255, index=w1257) -> (element=w1256:string)
                      n807 = Fract/Exp String To Number(string=w1256) -> (number=w1253:dbl)  [unwired: 3 in, 1 out]
                    }
                    n808 = Array To Cluster(array=w1235) -> (cluster=w1234:T10)
                    n809 = Unbundle(w1234) -> ("[0]"=w1236:dbl, "[1]"=w1237:dbl, "[2]"=w1238:dbl, "[3]"=w1241:dbl, "[4]"=w1242:dbl, "[5]"=w1243:dbl)  [unwired: 3 out]
                    n810 = case shown="0, Default" w1241 {
                      tunnel: [enum16{"Left", "Right"}."Right" enum16{"Left", "Right"}."Left"] -> w1244
                      frame 0, Default {
                      }
                      frame 1 {
                      }
                    }
                    n811 = case shown="0, Default" w1242 {
                      tunnel: [enum16{"Forward", "Backward"}."Forward" enum16{"Forward", "Backward"}."Backward"] -> w1246
                      frame 0, Default {
                      }
                      frame 1 {
                      }
                    }
                    n812 = case shown="0, Default" w1243 {
                      tunnel: [enum16{"Up", "Down"}."Down" enum16{"Up", "Down"}."Up"] -> w1245
                      frame 0, Default {
                      }
                      frame 1 {
                      }
                    }
                    n813 = Bundle("[0]"=w1236, "[1]"=w1237, "[2]"=w1238) -> (w1239:cluster{"[0]":dbl, "[1]":dbl, "[2]":dbl})  [unwired: 1 in]
                    n814 = Cluster To Array(cluster=w1239) -> (array=w1240:dbl[])
                    n815 = local write "Steps(mm)"(w1240) -> ()
                    n816 = local write "X axis"(w1244) -> ()
                    n817 = local write "Z axis"(w1245) -> ()
                    n818 = local write "Y axis"(w1246) -> ()
                  }
                  frame #1 {
                    n819 = local write "Operation Done"("Steps Set") -> ()
                  }
                }
              }
              frame "Set Count" {
                n820 = flat-sequence {
                  frame #0 {
                    n821 = local read "Current Sequence"() -> (w1264:string[])
                    n822 = Index Array(array=w1264, index=1) -> (element=w1263:string)
                    n823 = Fract/Exp String To Number(string=w1263) -> (number=w1265:dbl)  [unwired: 3 in, 1 out]
                    n824 = local write "Count"(w1265) -> ()
                  }
                  frame #1 {
                    n825 = local write "Operation Done"("Count Set") -> ()
                  }
                }
              }
              frame "SensStage Move" {
                n826 = local read "Activate Sequence?"() -> (w1272:bool)
                n827 = local read "Move Abs S"() -> (w1276:bool)
                n828 = case shown="True" w1272 {
                  tunnel: "error in 4" -> [w1277 w1279]
                  tunnel: [w1277 w1278] -> w1270
                  frame False {
                  }
                  frame True {
                    n829 = local read "Current Sequence"() -> (w1281:string[])
                    n830 = Index Array(array=w1281, index=1) -> (element=w1280:string)
                    n831 = case shown="\"MoveAbs\", Default" w1280 {
                      tunnel: w1279 -> [w1287 w1327]
                      tunnel: [w1283 w1323] -> w1278
                      frame "MovRel" {
                        n832 = flat-sequence {
                          tunnel: [w1294] -> w1293
                          tunnel: [w1297] -> w1290
                          tunnel: w1287 -> [w1296]
                          tunnel: [w1295] -> w1286
                          tunnel: w1293 -> [w1308]
                          tunnel: [w1308] -> w1292
                          tunnel: w1290 -> [w1307]
                          tunnel: [w1307] -> w1289
                          tunnel: w1286 -> [w1301]
                          tunnel: [w1300] -> w1285
                          tunnel: w1292 -> [w1315]
                          tunnel: [w1315] -> w1291
                          tunnel: w1289 -> [w1314]
                          tunnel: [w1314] -> w1288
                          tunnel: w1285 -> [w1313]
                          tunnel: [w1312] -> w1284
                          tunnel: w1291 -> [w1322]
                          tunnel: w1288 -> [w1321]
                          tunnel: w1284 -> [w1320]
                          tunnel: [w1318] -> w1283
                          frame #0 {
                            n833 = local read "Axes to move S"() -> (w1297:string[])
                            n834 = local read "System no. S"() -> (w1294:i32)
                            n835 = call "VEL.vi"("System no."=w1294, "Axes to set"=w1297, "Velocity values"=dbl[] [2.0], "error in"=w1296) -> ("error out"=w1295:errorcluster)  [unwired: 14 in, 1 out]
                          }
                          frame #1 {
                            n836 = local read "Current Sequence"() -> (w1305:string[])
                            n837 = local write "Moving"(TRUE ("Moving")) -> ()
                            n838 = Index Array(array=w1305, index=2) -> (element=w1303:string)
                            n839 = Fract/Exp String To Number(string=w1303) -> (number=w1306:dbl)  [unwired: 3 in, 1 out]
                            n840 = Build Array(w1306) -> (w1302:dbl[])
                            n841 = call "MVR.vi"("System no."=w1308, "Axes to move"=w1307, "Position values"=w1302, "No.of digits"=i16 4, "error in"=w1301) -> ("error out"=w1300:errorcluster)  [unwired: 14 in]
                          }
                          frame #2 {
                            n842 = local write "Moving"(FALSE ("Moving")) -> ()
                            n843 = call "General wait for movement to stop.vi"("System no."=w1315, "Axes to wait for"=w1314, "Additional wait time, ms"=u32 500, "error in"=w1313) -> ("Stopped"=w1311:bool, "error out"=w1312:errorcluster)  [unwired: 14 in]
                            n844 = local write "Stopped"(w1311) -> ()
                          }
                          frame #3 {
                            n845 = call "POS?.vi"("System no."=w1322, "Axes to query"=w1321, "error in"=w1320) -> ("Position"=w1319:dbl[], "error out"=w1318:errorcluster)  [unwired: 15 in]
                            n846 = local write "SensorStage - Zaxis"(w1319) -> ()
                            n847 = local write "Move Rel S"(FALSE ("Move Rel S")) -> ()
                          }
                        }
                      }
                      frame "MoveAbs", Default {
                        n848 = flat-sequence {
                          tunnel: [w1334] -> w1333
                          tunnel: [w1337] -> w1330
                          tunnel: w1327 -> [w1336]
                          tunnel: [w1335] -> w1326
                          tunnel: w1333 -> [w1348]
                          tunnel: [w1348] -> w1332
                          tunnel: w1330 -> [w1347]
                          tunnel: [w1347] -> w1329
                          tunnel: w1326 -> [w1341]
                          tunnel: [w1340] -> w1325
                          tunnel: w1332 -> [w1355]
                          tunnel: [w1355] -> w1331
                          tunnel: w1329 -> [w1354]
                          tunnel: [w1354] -> w1328
                          tunnel: w1325 -> [w1353]
                          tunnel: [w1352] -> w1324
                          tunnel: w1331 -> [w1362]
                          tunnel: w1328 -> [w1361]
                          tunnel: w1324 -> [w1359]
                          tunnel: [w1358] -> w1323
                          frame #0 {
                            n849 = local read "Axes to move S"() -> (w1337:string[])
                            n850 = local read "System no. S"() -> (w1334:i32)
                            n851 = call "VEL.vi"("System no."=w1334, "Axes to set"=w1337, "Velocity values"=dbl[] [2.0], "error in"=w1336) -> ("error out"=w1335:errorcluster)  [unwired: 14 in, 1 out]
                          }
                          frame #1 {
                            n852 = local read "Current Sequence"() -> (w1345:string[])
                            n853 = local write "Moving"(TRUE ("Moving")) -> ()
                            n854 = Index Array(array=w1345, index=2) -> (element=w1343:string)
                            n855 = Fract/Exp String To Number(string=w1343) -> (number=w1344:dbl)  [unwired: 3 in, 1 out]
                            n856 = Build Array(w1344) -> (w1342:dbl[])
                            n857 = call "MOV.vi"("System no."=w1348, "Axes to move"=w1347, "Position values"=w1342, "No.of digits"=i16 4, "error in"=w1341) -> ("error out"=w1340:errorcluster)  [unwired: 14 in]
                          }
                          frame #2 {
                            n858 = call "General wait for movement to stop.vi"("System no."=w1355, "Axes to wait for"=w1354, "Additional wait time, ms"=u32 500, "error in"=w1353) -> ("Stopped"=w1351:bool, "error out"=w1352:errorcluster)  [unwired: 14 in]
                            n859 = local write "Stopped"(w1351) -> ()
                            n860 = local write "Moving"(FALSE ("Moving")) -> ()
                          }
                          frame #3 {
                            n861 = call "POS?.vi"("System no."=w1362, "Axes to query"=w1361, "error in"=w1359) -> ("Position"=w1360:dbl[], "error out"=w1358:errorcluster)  [unwired: 15 in]
                            n862 = local write "SensorStage - Zaxis"(w1360) -> ()
                            n863 = local write "Move Abs S"(FALSE ("Move Abs S")) -> ()
                          }
                        }
                      }
                    }
                  }
                }
                "error out 7" <- w1270
                n864 = local read "Move Rel S"() -> (w1275:bool)
                n865 = case shown="True" w1275 {
                  tunnel: "error in 4" -> [w1363 w1368]
                  tunnel: [w1363 w1364] -> w1273
                  frame False {
                  }
                  frame True {
                    n866 = flat-sequence {
                      tunnel: [w1375] -> w1374
                      tunnel: [w1378] -> w1371
                      tunnel: w1368 -> [w1377]
                      tunnel: [w1376] -> w1367
                      tunnel: w1374 -> [w1385]
                      tunnel: [w1385] -> w1373
                      tunnel: w1371 -> [w1383]
                      tunnel: [w1383] -> w1370
                      tunnel: w1367 -> [w1382]
                      tunnel: [w1381] -> w1366
                      tunnel: w1373 -> [w1392]
                      tunnel: [w1392] -> w1372
                      tunnel: w1370 -> [w1391]
                      tunnel: [w1391] -> w1369
                      tunnel: w1366 -> [w1390]
                      tunnel: [w1389] -> w1365
                      tunnel: w1372 -> [w1399]
                      tunnel: w1369 -> [w1397]
                      tunnel: w1365 -> [w1396]
                      tunnel: [w1395] -> w1364
                      frame #0 {
                        n867 = local read "Axes to move S"() -> (w1378:string[])
                        n868 = local read "System no. S"() -> (w1375:i32)
                        n869 = call "VEL.vi"("System no."=w1375, "Axes to set"=w1378, "Velocity values"=dbl[] [2.0], "error in"=w1377) -> ("error out"=w1376:errorcluster)  [unwired: 14 in, 1 out]
                      }
                      frame #1 {
                        n870 = local write "Moving"(TRUE ("Moving")) -> ()
                        n871 = call "MVR.vi"("System no."=w1385, "Axes to move"=w1383, "Position values"="Steps to move-S", "No.of digits"=i16 4, "error in"=w1382) -> ("error out"=w1381:errorcluster)  [unwired: 14 in]
                      }
                      frame #2 {
                        n872 = call "General wait for movement to stop.vi"("System no."=w1392, "Axes to wait for"=w1391, "Additional wait time, ms"=u32 500, "error in"=w1390) -> ("Stopped"=w1388:bool, "error out"=w1389:errorcluster)  [unwired: 14 in]
                        n873 = local write "Moving"(FALSE ("Moving")) -> ()
                        n874 = local write "Stopped"(w1388) -> ()
                      }
                      frame #3 {
                        n875 = call "POS?.vi"("System no."=w1399, "Axes to query"=w1397, "error in"=w1396) -> ("Position"=w1398:dbl[], "error out"=w1395:errorcluster)  [unwired: 15 in]
                        n876 = local write "SensorStage - Zaxis"(w1398) -> ()
                        n877 = local write "Move Rel S"(FALSE ("Move Rel S")) -> ()
                      }
                    }
                  }
                }
                "error out 6" <- w1273
                n878 = case shown="True" w1276 {
                  tunnel: "error in 4" -> [w1400 w1402]
                  tunnel: [w1400 w1401] -> w1274
                  frame False {
                  }
                  frame True {
                    n879 = flat-sequence {
                      tunnel: [w1412] -> w1411
                      tunnel: [w1415] -> w1408
                      tunnel: w1402 -> [w1414]
                      tunnel: [w1413] -> w1405
                      tunnel: w1411 -> [w1422]
                      tunnel: [w1422] -> w1410
                      tunnel: w1408 -> [w1420]
                      tunnel: [w1420] -> w1407
                      tunnel: w1405 -> [w1419]
                      tunnel: [w1418] -> w1404
                      tunnel: w1410 -> [w1429]
                      tunnel: [w1429] -> w1409
                      tunnel: w1407 -> [w1428]
                      tunnel: [w1428] -> w1406
                      tunnel: w1404 -> [w1427]
                      tunnel: [w1426] -> w1403
                      tunnel: w1409 -> [w1436]
                      tunnel: w1406 -> [w1435]
                      tunnel: [w1433] -> w1401
                      tunnel: w1403 -> [w1432]
                      frame #0 {
                        n880 = local read "System no. S"() -> (w1412:i32)
                        n881 = local read "Axes to move S"() -> (w1415:string[])
                        n882 = call "VEL.vi"("System no."=w1412, "Axes to set"=w1415, "Velocity values"=dbl[] [2.0], "error in"=w1414) -> ("error out"=w1413:errorcluster)  [unwired: 14 in, 1 out]
                      }
                      frame #1 {
                        n883 = local write "Moving"(TRUE ("Moving")) -> ()
                        n884 = call "MOV.vi"("System no."=w1422, "Axes to move"=w1420, "Position values"="Position to move-S", "No.of digits"=i16 4, "error in"=w1419) -> ("error out"=w1418:errorcluster)  [unwired: 14 in]
                      }
                      frame #2 {
                        n885 = local write "Moving"(FALSE ("Moving")) -> ()
                        n886 = call "General wait for movement to stop.vi"("System no."=w1429, "Axes to wait for"=w1428, "Additional wait time, ms"=u32 500, "error in"=w1427) -> ("Stopped"=w1425:bool, "error out"=w1426:errorcluster)  [unwired: 14 in]
                        n887 = local write "Stopped"(w1425) -> ()
                      }
                      frame #3 {
                        n888 = call "POS?.vi"("System no."=w1436, "Axes to query"=w1435, "error in"=w1432) -> ("Position"=w1434:dbl[], "error out"=w1433:errorcluster)  [unwired: 15 in]
                        n889 = local write "SensorStage - Zaxis"(w1434) -> ()
                        n890 = local write "Move Abs S"(FALSE ("Move Abs S")) -> ()
                      }
                    }
                  }
                }
                "error out 5" <- w1274
              }
              frame "YaxisStage Move" {
                n891 = local read "Activate Sequence?"() -> (w1441:bool)
                n892 = local read "Move Abs Y"() -> (w1444:bool)
                n893 = local read "Move Rel Y"() -> (w1443:bool)
                n894 = case shown="True" w1441 {
                  tunnel: [w1447 w1449] -> w1438
                  tunnel: "error in" -> [w1447 w1448]
                  frame False {
                  }
                  frame True {
                    n895 = local read "Current Sequence"() -> (w1451:string[])
                    n896 = Index Array(array=w1451, index=1) -> (element=w1450:string)
                    n897 = case shown="\"MoveRel\"" w1450 {
                      tunnel: [w1453 w1496] -> w1449
                      tunnel: w1448 -> [w1454 w1495]
                      frame "MoveRel" {
                        n898 = flat-sequence {
                          tunnel: [w1464] -> w1463
                          tunnel: [w1468] -> w1462
                          tunnel: [w1467] -> w1461
                          tunnel: w1454 -> [w1465]
                          tunnel: w1463 -> [w1470]
                          tunnel: w1462 -> [w1471]
                          tunnel: [w1470] -> w1460
                          tunnel: [w1471] -> w1459
                          tunnel: w1461 -> [w1473]
                          tunnel: [w1474] -> w1458
                          tunnel: w1460 -> [w1482]
                          tunnel: w1459 -> [w1481]
                          tunnel: [w1482] -> w1457
                          tunnel: [w1481] -> w1456
                          tunnel: w1458 -> [w1480]
                          tunnel: [w1479] -> w1455
                          tunnel: w1457 -> [w1493]
                          tunnel: w1456 -> [w1492]
                          tunnel: w1455 -> [w1491]
                          tunnel: [w1490] -> w1453
                          frame #0 {
                            n899 = local read "System no.Y"() -> (w1464:i32)
                            n900 = local read "Axes to move Y"() -> (w1468:string[])
                            n901 = call "VEL.vi"("System no."=w1464, "Axes to set"=w1468, "Velocity values"=dbl[] [5.0], "error in"=w1465) -> ("error out"=w1467:errorcluster)  [unwired: 14 in, 1 out]
                          }
                          frame #1 {
                            n902 = local read "Current Sequence"() -> (w1477:string[])
                            n903 = Index Array(array=w1477, index=2) -> (element=w1476:string)
                            n904 = Fract/Exp String To Number(string=w1476) -> (number=w1475:dbl)  [unwired: 3 in, 1 out]
                            n905 = Build Array(w1475) -> (w1472:dbl[])
                            n906 = call "MVR.vi"("System no."=w1470, "Axes to move"=w1471, "Position values"=w1472, "No.of digits"=i16 4, "error in"=w1473) -> ("error out"=w1474:errorcluster)  [unwired: 14 in]
                          }
                          frame #2 {
                            n907 = call "General wait for movement to stop.vi"("System no."=w1482, "Axes to wait for"=w1481, "Additional wait time, ms"=u32 500, "error in"=w1480) -> ("error out"=w1479:errorcluster)  [unwired: 14 in, 1 out]
                          }
                          frame #3 {
                            w1485 = FALSE ("Sensors Active?")
                            n908 = call "POS?.vi"("System no."=w1493, "Axes to query"=w1492, "error in"=w1491) -> ("Position"=w1494:dbl[], "error out"=w1490:errorcluster)  [unwired: 15 in]
                            n909 = local write "Yaxis Stage"(w1494) -> ()
                            n910 = local read "Port for ED33"() -> (w1487:refnum<visa-resource-name>)
                            n911 = Not(x=w1485) -> (.not. x?=w1486:bool)
                            n912 = call "Sensor_Read.vi"("Sensors Active?"=w1485, "ED33 Active?"=w1486, "Port ED33"=w1487) -> ("ED33_output"=w1488:string[][])  [unwired: 7 in, 1 out]
                            n913 = Index Array(array=w1488, index (row)=0 ("disabled index (col)")) -> (element=w1484:string[])  [unwired: 1 in]
                            n914 = local write "Sensor Output"(w1484) -> ()
                          }
                        }
                      }
                      frame "MoveAbs", Default {
                        n915 = flat-sequence {
                          tunnel: [w1506] -> w1505
                          tunnel: [w1510] -> w1504
                          tunnel: [w1509] -> w1499
                          tunnel: w1495 -> [w1507]
                          tunnel: w1505 -> [w1514]
                          tunnel: w1504 -> [w1513]
                          tunnel: [w1514] -> w1503
                          tunnel: [w1513] -> w1502
                          tunnel: w1499 -> [w1512]
                          tunnel: [w1511] -> w1498
                          tunnel: w1503 -> [w1523]
                          tunnel: w1502 -> [w1522]
                          tunnel: [w1523] -> w1501
                          tunnel: [w1522] -> w1500
                          tunnel: w1498 -> [w1521]
                          tunnel: [w1520] -> w1497
                          tunnel: w1501 -> [w1534]
                          tunnel: w1500 -> [w1533]
                          tunnel: w1497 -> [w1532]
                          tunnel: [w1531] -> w1496
                          frame #0 {
                            n916 = local read "System no.Y"() -> (w1506:i32)
                            n917 = local read "Axes to move Y"() -> (w1510:string[])
                            n918 = call "VEL.vi"("System no."=w1506, "Axes to set"=w1510, "Velocity values"=dbl[] [5.0], "error in"=w1507) -> ("error out"=w1509:errorcluster)  [unwired: 14 in, 1 out]
                          }
                          frame #1 {
                            n919 = local read "Current Sequence"() -> (w1518:string[])
                            n920 = Index Array(array=w1518, index=2) -> (element=w1517:string)
                            n921 = Fract/Exp String To Number(string=w1517) -> (number=w1516:dbl)  [unwired: 3 in, 1 out]
                            n922 = Build Array(w1516) -> (w1515:dbl[])
                            n923 = call "MOV.vi"("System no."=w1514, "Axes to move"=w1513, "Position values"=w1515, "error in"=w1512) -> ("error out"=w1511:errorcluster)  [unwired: 15 in]
                          }
                          frame #2 {
                            n924 = call "General wait for movement to stop.vi"("System no."=w1523, "Axes to wait for"=w1522, "Additional wait time, ms"=u32 500, "error in"=w1521) -> ("error out"=w1520:errorcluster)  [unwired: 14 in, 1 out]
                          }
                          frame #3 {
                            w1529 = FALSE ("Sensors Active?")
                            n925 = call "POS?.vi"("System no."=w1534, "Axes to query"=w1533, "error in"=w1532) -> ("Position"=w1535:dbl[], "error out"=w1531:errorcluster)  [unwired: 15 in]
                            n926 = local write "Yaxis Stage"(w1535) -> ()
                            n927 = local read "Port for ED33"() -> (w1527:refnum<visa-resource-name>)
                            n928 = Not(x=w1529) -> (.not. x?=w1528:bool)
                            n929 = call "Sensor_Read.vi"("Sensors Active?"=w1529, "ED33 Active?"=w1528, "Port ED33"=w1527) -> ("ED33_output"=w1526:string[][])  [unwired: 7 in, 1 out]
                            n930 = Index Array(array=w1526, index (row)=0 ("disabled index (col)")) -> (element=w1530:string[])  [unwired: 1 in]
                            n931 = local write "Sensor Output"(w1530) -> ()
                          }
                        }
                      }
                    }
                  }
                }
                "error out 3" <- w1438
                n932 = case shown="True" w1443 {
                  tunnel: [w1536 w1538] -> w1439
                  tunnel: "error in" -> [w1536 w1537]
                  frame False {
                  }
                  frame True {
                    n933 = flat-sequence {
                      tunnel: [w1552] -> w1547
                      tunnel: [w1548] -> w1546
                      tunnel: [w1551] -> w1545
                      tunnel: w1537 -> [w1549]
                      tunnel: w1547 -> [w1554]
                      tunnel: w1546 -> [w1555]
                      tunnel: w1545 -> [w1558]
                      tunnel: [w1557] -> w1544
                      tunnel: [w1555] -> w1542
                      tunnel: [w1554] -> w1540
                      tunnel: w1544 -> [w1566]
                      tunnel: [w1565] -> w1543
                      tunnel: w1542 -> [w1562]
                      tunnel: [w1562] -> w1541
                      tunnel: w1540 -> [w1561]
                      tunnel: [w1561] -> w1539
                      tunnel: w1543 -> [w1578]
                      tunnel: w1541 -> [w1575]
                      tunnel: w1539 -> [w1574]
                      tunnel: [w1573] -> w1538
                      frame #0 {
                        n934 = local read "System no.Y"() -> (w1548:i32)
                        n935 = local read "Axes to move Y"() -> (w1552:string[])
                        n936 = call "VEL.vi"("System no."=w1548, "Axes to set"=w1552, "Velocity values"=dbl[] [5.0], "error in"=w1549) -> ("error out"=w1551:errorcluster)  [unwired: 14 in, 1 out]
                      }
                      frame #1 {
                        n937 = local write "Moving"(TRUE ("Moving")) -> ()
                        n938 = call "MVR.vi"("System no."=w1555, "Axes to move"=w1554, "Position values"="Steps to move-Y", "No.of digits"=i16 4, "error in"=w1558) -> ("error out"=w1557:errorcluster)  [unwired: 14 in]
                      }
                      frame #2 {
                        n939 = call "General wait for movement to stop.vi"("System no."=w1562, "Axes to wait for"=w1561, "Additional wait time, ms"=u32 500, "error in"=w1566) -> ("Stopped"=w1564:bool, "error out"=w1565:errorcluster)  [unwired: 14 in]
                        n940 = local write "Moving"(FALSE ("Moving")) -> ()
                        n941 = local write "Stopped"(w1564) -> ()
                      }
                      frame #3 {
                        w1568 = FALSE ("Sensors Active?")
                        n942 = call "POS?.vi"("System no."=w1575, "Axes to query"=w1574, "error in"=w1578) -> ("Position"=w1577:dbl[], "error out"=w1573:errorcluster)  [unwired: 15 in]
                        n943 = local write "Move Rel Y"(FALSE ("Move Rel")) -> ()
                        n944 = local write "Yaxis Stage"(w1577) -> ()
                        n945 = local read "Port for ED33"() -> (w1570:refnum<visa-resource-name>)
                        n946 = Not(x=w1568) -> (.not. x?=w1569:bool)
                        n947 = call "Sensor_Read.vi"("Sensors Active?"=w1568, "ED33 Active?"=w1569, "Port ED33"=w1570) -> ("ED33_output"=w1571:string[][])  [unwired: 7 in, 1 out]
                        n948 = Index Array(array=w1571, index (row)=0 ("disabled index (col)")) -> (element=w1567:string[])  [unwired: 1 in]
                        n949 = local write "Sensor Output"(w1567) -> ()
                      }
                    }
                  }
                }
                "error out 2" <- w1439
                n950 = case shown="True" w1444 {
                  tunnel: [w1579 w1581] -> w1440
                  tunnel: "error in" -> [w1579 w1580]
                  frame False {
                  }
                  frame True {
                    n951 = flat-sequence {
                      tunnel: [w1594] -> w1590
                      tunnel: [w1591] -> w1589
                      tunnel: [w1595] -> w1588
                      tunnel: w1580 -> [w1592]
                      tunnel: [w1597] -> w1587
                      tunnel: [w1598] -> w1586
                      tunnel: [w1599] -> w1585
                      tunnel: w1590 -> [w1598]
                      tunnel: w1589 -> [w1597]
                      tunnel: w1588 -> [w1596]
                      tunnel: w1587 -> [w1606]
                      tunnel: w1586 -> [w1605]
                      tunnel: [w1606] -> w1584
                      tunnel: [w1605] -> w1583
                      tunnel: [w1604] -> w1582
                      tunnel: w1585 -> [w1603]
                      tunnel: w1584 -> [w1621]
                      tunnel: w1583 -> [w1620]
                      tunnel: w1582 -> [w1619]
                      tunnel: [w1616] -> w1581
                      frame #0 {
                        n952 = local read "System no.Y"() -> (w1591:i32)
                        n953 = local read "Axes to move Y"() -> (w1594:string[])
                        n954 = call "VEL.vi"("System no."=w1591, "Axes to set"=w1594, "Velocity values"=dbl[] [5.0], "error in"=w1592) -> ("error out"=w1595:errorcluster)  [unwired: 14 in, 1 out]
                      }
                      frame #1 {
                        n955 = local write "Moving"(TRUE ("Moving")) -> ()
                        n956 = call "MOV.vi"("System no."=w1597, "Axes to move"=w1598, "Position values"="Position to move-Y", "No.of digits"=i16 4, "error in"=w1596) -> ("error out"=w1599:errorcluster)  [unwired: 14 in]
                      }
                      frame #2 {
                        n957 = local write "Moving"(FALSE ("Moving")) -> ()
                        n958 = call "General wait for movement to stop.vi"("System no."=w1606, "Axes to wait for"=w1605, "Additional wait time, ms"=u32 500, "error in"=w1603) -> ("Stopped"=w1608:bool, "error out"=w1604:errorcluster)  [unwired: 14 in]
                        n959 = local write "Stopped"(w1608) -> ()
                      }
                      frame #3 {
                        w1614 = FALSE ("Sensors Active?")
                        n960 = call "POS?.vi"("System no."=w1621, "Axes to query"=w1620, "error in"=w1619) -> ("Position"=→"Yaxis Stage":dbl[], "error out"=w1616:errorcluster)  [unwired: 15 in]
                        n961 = local write "Move Abs Y"(FALSE ("Move To")) -> ()
                        n962 = local read "Port for ED33"() -> (w1612:refnum<visa-resource-name>)
                        n963 = Not(x=w1614) -> (.not. x?=w1613:bool)
                        n964 = call "Sensor_Read.vi"("Sensors Active?"=w1614, "ED33 Active?"=w1613, "Port ED33"=w1612) -> ("ED33_output"=w1611:string[][])  [unwired: 7 in, 1 out]
                        n965 = Index Array(array=w1611, index (row)=0 ("disabled index (col)")) -> (element=w1615:string[])  [unwired: 1 in]
                        n966 = local write "Sensor Output"(w1615) -> ()
                      }
                    }
                  }
                }
                "error out" <- w1440
              }
              frame "Wait", Default {
                n967 = Wait (ms)(milliseconds to wait=50) -> ()  [unwired: 1 out]
                n968 = local write "Current Status"("Waiting for next instruction" ("Status")) -> ()
              }
              frame "Write Pole" {
                n969 = local read "Current Sequence"() -> (w1632:string[])
                n970 = local read "Port for Powersupply"() -> (w1630:refnum<visa-resource-name>)
                n971 = local read "Port for Write Head"() -> (w1631:refnum<visa-resource-name>)
                n972 = call "Write Pole.vi"("Fehler (Eingang)"=w1629, "array"=w1632, "Port for write head"=w1631, "Port for Powersupply"=w1630) -> ("Fehler (Ausgang)"=w1628:errorcluster)
              }
            }
          }
          frame Error {
            n973 = Unbundle(w1635) -> ("source"=w1634:string)  [unwired: 2 out]
            n974 = One Button Dialog(message=w1634) -> (true=w1638:bool)  [unwired: 1 in]
            n975 = local write "Stopped"(w1638) -> ()
            n976 = local write "Stop Program"(w1638) -> ()
            n977 = local write "Current Status"("Force stop due to error" ("Status")) -> ()
          }
        }
        n978 = local read "Stop Program"() -> (w33:bool)
        n979 = flat-sequence {
          tunnel: [w76] -> w40
          tunnel: w41 -> [w75]
          frame #0 {
            n980 = local read "Current Status"() -> (w77:string)
            n981 = case shown="\"Waiting for next instruction\"" w77 {
              selector: w77 -> [w79 _]
              tunnel: [w79 w80] -> w76
              tunnel: w75 -> [_ w80]
              frame "Pause", Default {
                n982 = local write "Current Status"("Waiting for next instruction" ("Status")) -> ()
              }
              frame "Waiting for next instruction" {
              }
            }
          }
        }
        n983 = case shown="False" w33 {
          frame False {
          }
          frame True {
            w69 = "" ("element")
            w72 = FALSE ("Moving")
            n984 = local read "Port for Powersupply"() -> (w59:refnum<visa-resource-name>)
            n985 = local read "Port for Write Head"() -> (w61:refnum<visa-resource-name>)
            n986 = local read "Port for Sensors"() -> (w60:refnum<visa-resource-name>)
            n987 = local read "Port for KOSY3"() -> (w58:refnum<visa-resource-name>)
            n988 = local write "Moving"(w72) -> ()
            n989 = local read "Port for ED33"() -> (w57:refnum<visa-resource-name>)
            n990 = Not(x=w72) -> (.not. x?=w73:bool)
            n991 = Initialize Array(w69) -> (w68:string[][])  [unwired: 2 in]
            n992 = Initialize Array(w69) -> (w70:string[])  [unwired: 1 in]
            n993 = local read "Error In"() -> (w62:errorcluster)
            n994 = local write "Stopped"(w73) -> ()
            n995 = global write "Global_Not-Aus.vi" "Not-Aus"(TRUE ("Not-Aus")) -> ()
            n996 = call "SubVI_Schliesse_COM_IF5_IF6.vi"("VISA resource name in"=w57, "error in"=w62) -> ("error out"=w63:errorcluster)  [unwired: 13 in]
            n997 = call "SubVI_Schliesse_COM_IF5_IF6.vi"("VISA resource name in"=w58, "error in"=w62) -> ("error out"=w64:errorcluster)  [unwired: 13 in]
            n998 = call "SubVI_Schliesse_COM_IF5_IF6.vi"("VISA resource name in"=w59, "error in"=w62) -> ("error out"=w67:errorcluster)  [unwired: 13 in]
            n999 = call "SubVI_Schliesse_COM_IF5_IF6.vi"("VISA resource name in"=w60, "error in"=w62) -> ("error out"=w66:errorcluster)  [unwired: 13 in]
            n1000 = call "SubVI_Schliesse_COM_IF5_IF6.vi"("VISA resource name in"=w61, "error in"=w62) -> ("error out"=w65:errorcluster)  [unwired: 13 in]
            n1001 = local write "Operation Done"("Program Stopped!!!" ("Status")) -> ()
            n1002 = local write "Sequence"(w68) -> ()
            n1003 = local write "Current Sequence"(w70) -> ()
            n1004 = local write "Error Out"(w63) -> ()
            n1005 = local write "Error Out"(w64) -> ()
            n1006 = local write "Error Out"(w67) -> ()
            n1007 = local write "Error Out"(w66) -> ()
            n1008 = local write "Error Out"(w65) -> ()
          }
        }
      }
    }
  }
  n1009 = local write "Error Out"(w1) -> ()
  n1010 = call <vilib>:"General Error Handler.vi"("error in (no error)"=w1) -> ()  [unwired: 10 in, 5 out]
